vi "METIS_main_005.vi"() -> ()   [LabVIEW 2020]
uses:
  <vilib>/Analysis/1siggen.llb/Ramp Pattern by Samples.vi
  <vilib>/DAQmx/write.llb/DAQmx Write (Analog DBL 1Chan 1Samp).vi
  <vilib>/DAQmx/miscellaneous.llb/DAQmx Fill In Error Info.vi
  <vilib>/DAQmx/create/channels.llb/DAQmx Create Channel (AO-Voltage-Basic).vi
  <userlib>/caLab/Private/Get_PV.vi
  <userlib>/caLab/Private/Put_I32-1D_PV-1D.vi
  <userlib>/caLab/Private/Put_I32_PV.vi
  <userlib>/caLab/Private/Put_DBL_PV.vi
  libraries/Newport ESP301/Newport ESP301.lvlib
  <vilib>/Analysis/NI_AALBase.lvlib
  <vilib>/ptbypt/NI_PtbyPt.lvlib
  libraries/ZaberTSeries/ZaberTSeries.lvlib
  <vilib>/Analysis/NI_AALPro.lvlib
  <vilib>/Utility/file.llb/Write Delimited Spreadsheet (string).vi
  <vilib>/Analysis/1siggen.llb/Ramp Pattern by Delta.vi
panel:
  out "String":string
  out "Waveform Chart":dbl(graph)
  in  "Tab Control":T1(tab)
  in  "delay_go":bool
  in  "delay_destination_fs":dbl=0.1 caption="Destination [fs]" step=1.0 format="%#.0f"
  in  "delay_destination_mm":dbl=0.1 caption="Destination [mm]"
  in  "delay_velocity":dbl caption="velocity [mm/s]"
  in  "delay_set_vel":bool
  in  "time_zero":dbl=1.0 caption="t0 [mm]"
  out "delay_pos_mm":dbl=1.0624 caption="Position [mm]" format="%08.4g"
  out "delay_pos_fs":dbl=416.2879908072938 caption="Time [fs]"
  in  "delay_set_t0":bool
  in  "delay_rel_mm_+":bool
  in  "delay_rel_mm_-":bool
  in  "delay_stepsize_mm":dbl=1.0 caption="step size [mm]"
  in  "delay_stepsize_fs":dbl=1.0 caption="step size [fs]"
  in  "delay_rel_fs_+":bool
  in  "delay_rel_fs_-":bool
  in  "pump_rel_+":bool
  in  "pump_rel_-":bool
  in  "pump_rel_delta":dbl=1.0 caption="step size [deg]"
  out "pump_position":dbl=1.0624 caption="Position [deg]"
  in  "probe_rel_+":bool
  in  "probe_rel_-":bool
  in  "probe_rel_delta":dbl=1.0 caption="step size [deg]"
  out "probe_position":dbl=416.2879908072938 caption="Position [deg]"
  out "zaber_Ypos":i32=2950 caption="Y"
  out "zaber_Xpos":i32=1955 caption="X"
  in  "mirr_rel":i32=1 caption="relative [steps]"
  in  "mirr_Y-":bool
  in  "mirr_Y+":bool
  in  "mirr_X+":bool
  in  "mirr_X-":bool
  in  "update_scale":bool
  in  "stop after":bool
  out "scan progress":dbl(slide) scale=0.0..1.0
  in  "delay_mode_select":enum32{"Discrete Scan", "Continous Scan"}(tab)
  in  "discr_scan_MRC?":bool caption="use MRC?"
  in  "delay_waypoints":string[][](table)
  in  "delay_speedpoints":string[][](table)
  in  "stop now":bool
  in  "start":bool
  in  "Scan Axis":T2(radio)
  out "Intensity Graph":dbl[][](graph)
  out "Ydata":cluster{"Ramp Pattern":dbl[], dbl[]}[](graph)
  in  "gauss_fit":bool
  out "center":dbl
  out "FWHM":dbl
  in  "center_cursors":bool
  in  "delay_set_t0 gauss":bool
  out "current parameter value [fs | deg | steps]":dbl
  out "i":i32 caption="current iteration"
  out "current exposure time":dbl
  in  "ADC Bit/Volt":dbl=627.0
  in  "zaber_patch":u8[](array[numeric])=[0, 1]
  in  "ESP Patch":i32[](array[numeric])=[3, 2, 1] min=1 max=3 step=1
  in  "ESP301 COM PORT":refnum<visa-resource-name>="COM5"
  in  "Serial Link (RS232)":enum16{"RS232", "USB"}(ring)
  in  "toADC":tag="Dev1/ao1"
  out "ESP error":errorcluster={"status"=TRUE, "code"=-1073807339, "source"="VISA Read in Newport ESP301.lvlib:Write Command and Read.vi->Newport ESP301.lvlib:Error Query.vi->Newport ESP301.lvlib:Initialize.vi->METIS_main_004.vi"}
  out "DAC error":errorcluster={"status"=TRUE, "code"=-200220, "source"="DAQmx Create Channel (AO-Voltage-Basic).vi:1870002<append>\n<B>Device Specified: </B>Dev3\n<B>Suggested Device(s): </B>Dev1\n\n<B>Task Name: </B>_unnamedTask<2>"}
  out "DAC_Voutput":dbl=5.25341140860948 caption="output voltage"
  in  "toMRC":tag="Dev1/ao0"
  in  "zaber_VISA":refnum<visa-resource-name>="COM7"
  out "zaber_error":errorcluster
  in  "main_close":bool
  # "Pump Waveplate"
  # "Delaystage"
  # "Zaber Mirror"
  # "Probe Waveplate"
  # "Delaystage"
  # "Pump Waveplate"
  # "Probe Waveplate"
  # "X"
  # "Y"
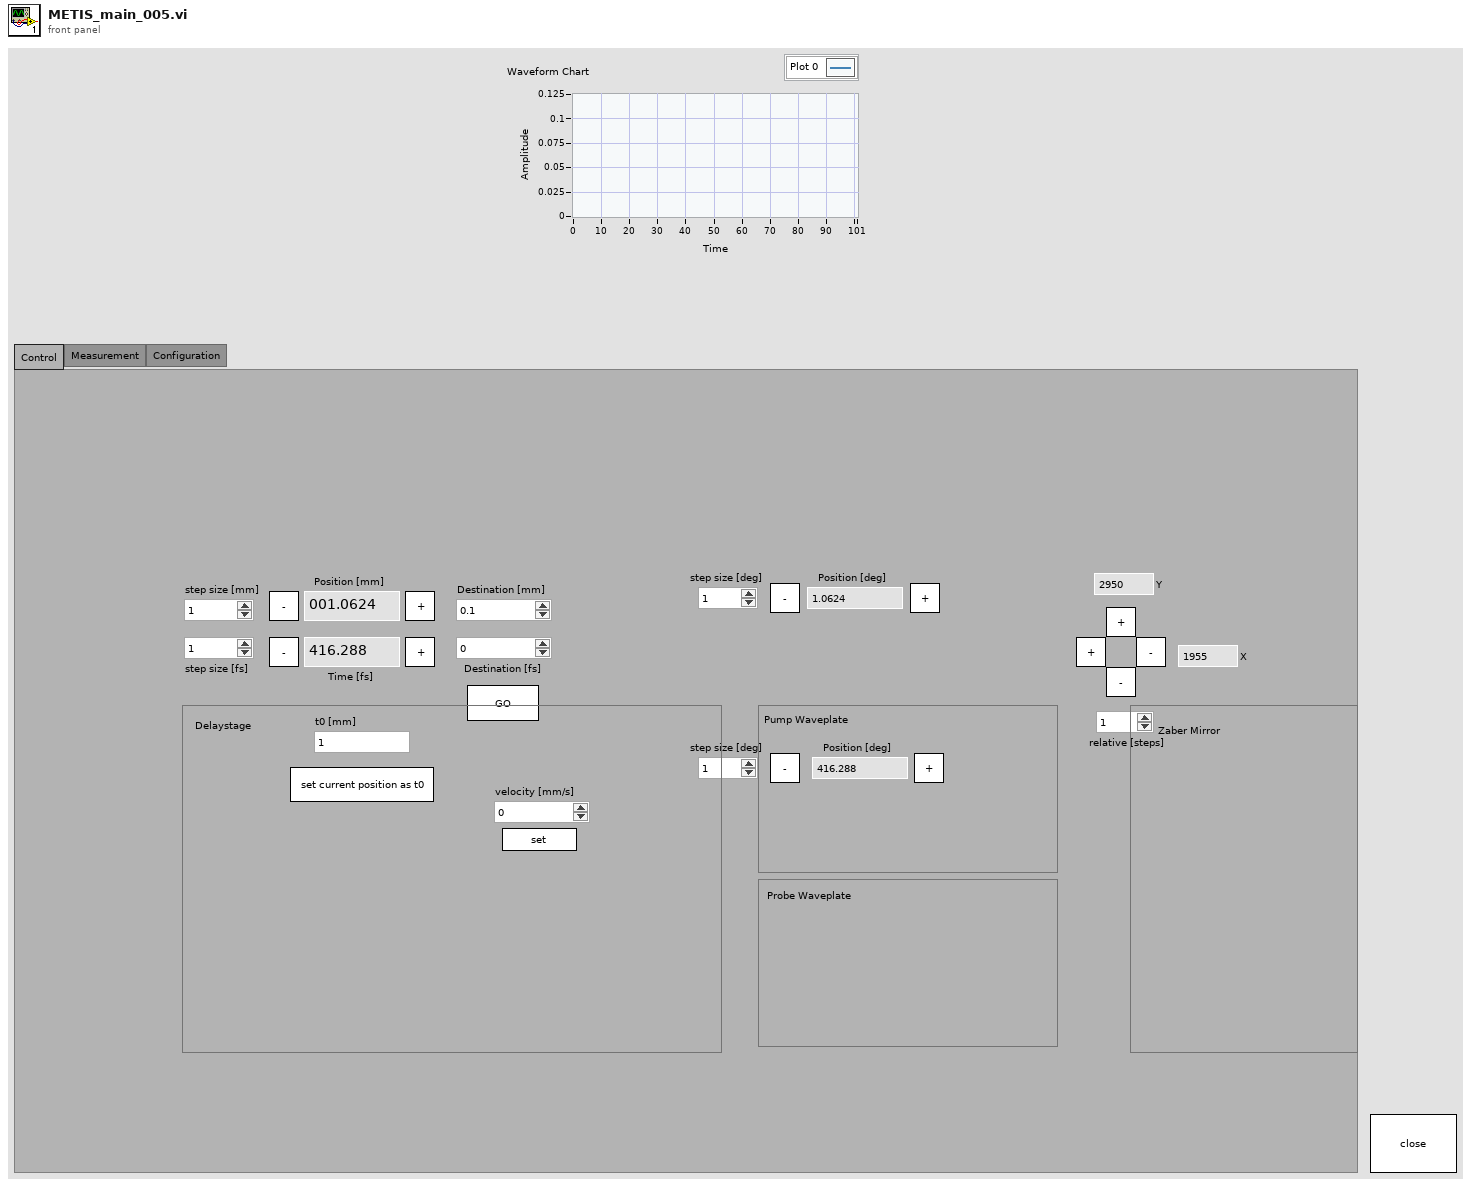
[diagram p1: front panel]
types:
  T1 = enum32{"Control", "Measurement", "Configuration"}
  T2 = enum32{"Item 0", "Item 1", "Radio Selection 3", "Radio Selection 4", "Radio Selection 5"}
  T3 = cluster{"ESP_cmd":refnum<queue>, "DAC_cmd":refnum<queue>, "meas_cmd":refnum<queue>, "zaber_cmd":refnum<queue>}
  T4 = cluster{"ESP_data":refnum<queue>, "dev2_data":refnum<queue>}
  T5 = cluster{"Axis 1":dbl, "Axis 2":dbl, "Axis 3":dbl}
  T6 = typedef "LVCursorListTypeDef.ctl" = cluster{"Name":string, "Color":u32, "Style":u8, "Point Style":u8, "Name Visible":bool, "Allow Drag":bool, "Cursor Mode":u32, "Plot":i32, "Index":i32, "Position":cluster{"X":dbl, "Y":dbl}, "X Scale":u32, "Y Scale":u32, "Watch Plots":i32[], "Watch All Plots":bool, "Plot Area":i32, "Label Offset":cluster{"X":dbl, "Y":dbl}}[]
  T7 = cluster{"Name":string, "Color":u32, "Style":u8, "Point Style":u8, "Name Visible":bool, "Allow Drag":bool, "Cursor Mode":u32, "Plot":i32, "Index":i32, "Position":cluster{"X":dbl, "Y":dbl}, "X Scale":u32, "Y Scale":u32, "Watch Plots":i32[], "Watch All Plots":bool, "Plot Area":i32, "Label Offset":cluster{"X":dbl, "Y":dbl}}
  T8 = cluster{"Name":string, "Color":u32, "Style":u8, "Point Style":u8, "Name Visible":bool, "Allow Drag":bool, "Cursor Mode":u32, "Plot":i32, "Index":i32, "Position":cluster{"X":dbl, "Y":dbl}, "X Scale":u32, "Y Scale":u32, "Watch Plots":i32[], "Watch All Plots":bool, "Plot Area":i32, "Label Offset":cluster{"X":dbl, "Y":dbl}}[]
  T9 = cluster{"Axis1 moving":bool, "Axis2 moving":bool, "Axis3 moving":bool, "Axis4 moving":bool, "Motor Power of at least one axis":bool, "Reserved":bool, "Reserved":bool, "Reserved":bool, "Axis5 moving 2":bool, "Axis6 moving 2":bool, "Reserved":bool, "Reserved":bool, "Motor Power of at least one axis":bool, "Reserved":bool, "Reserved":bool, "Reserved":bool}
  T10 = cluster{"Position (units)":dbl, "Position (units)":dbl, "Position (units)":dbl}
  T11 = cluster{"mirr_X# 4":u8, "Command":u8, dbl, "Response Count":i32}
  T12 = cluster{"mirr_X# 4":u8, "Command":u8, i32, "Response Count":i32}
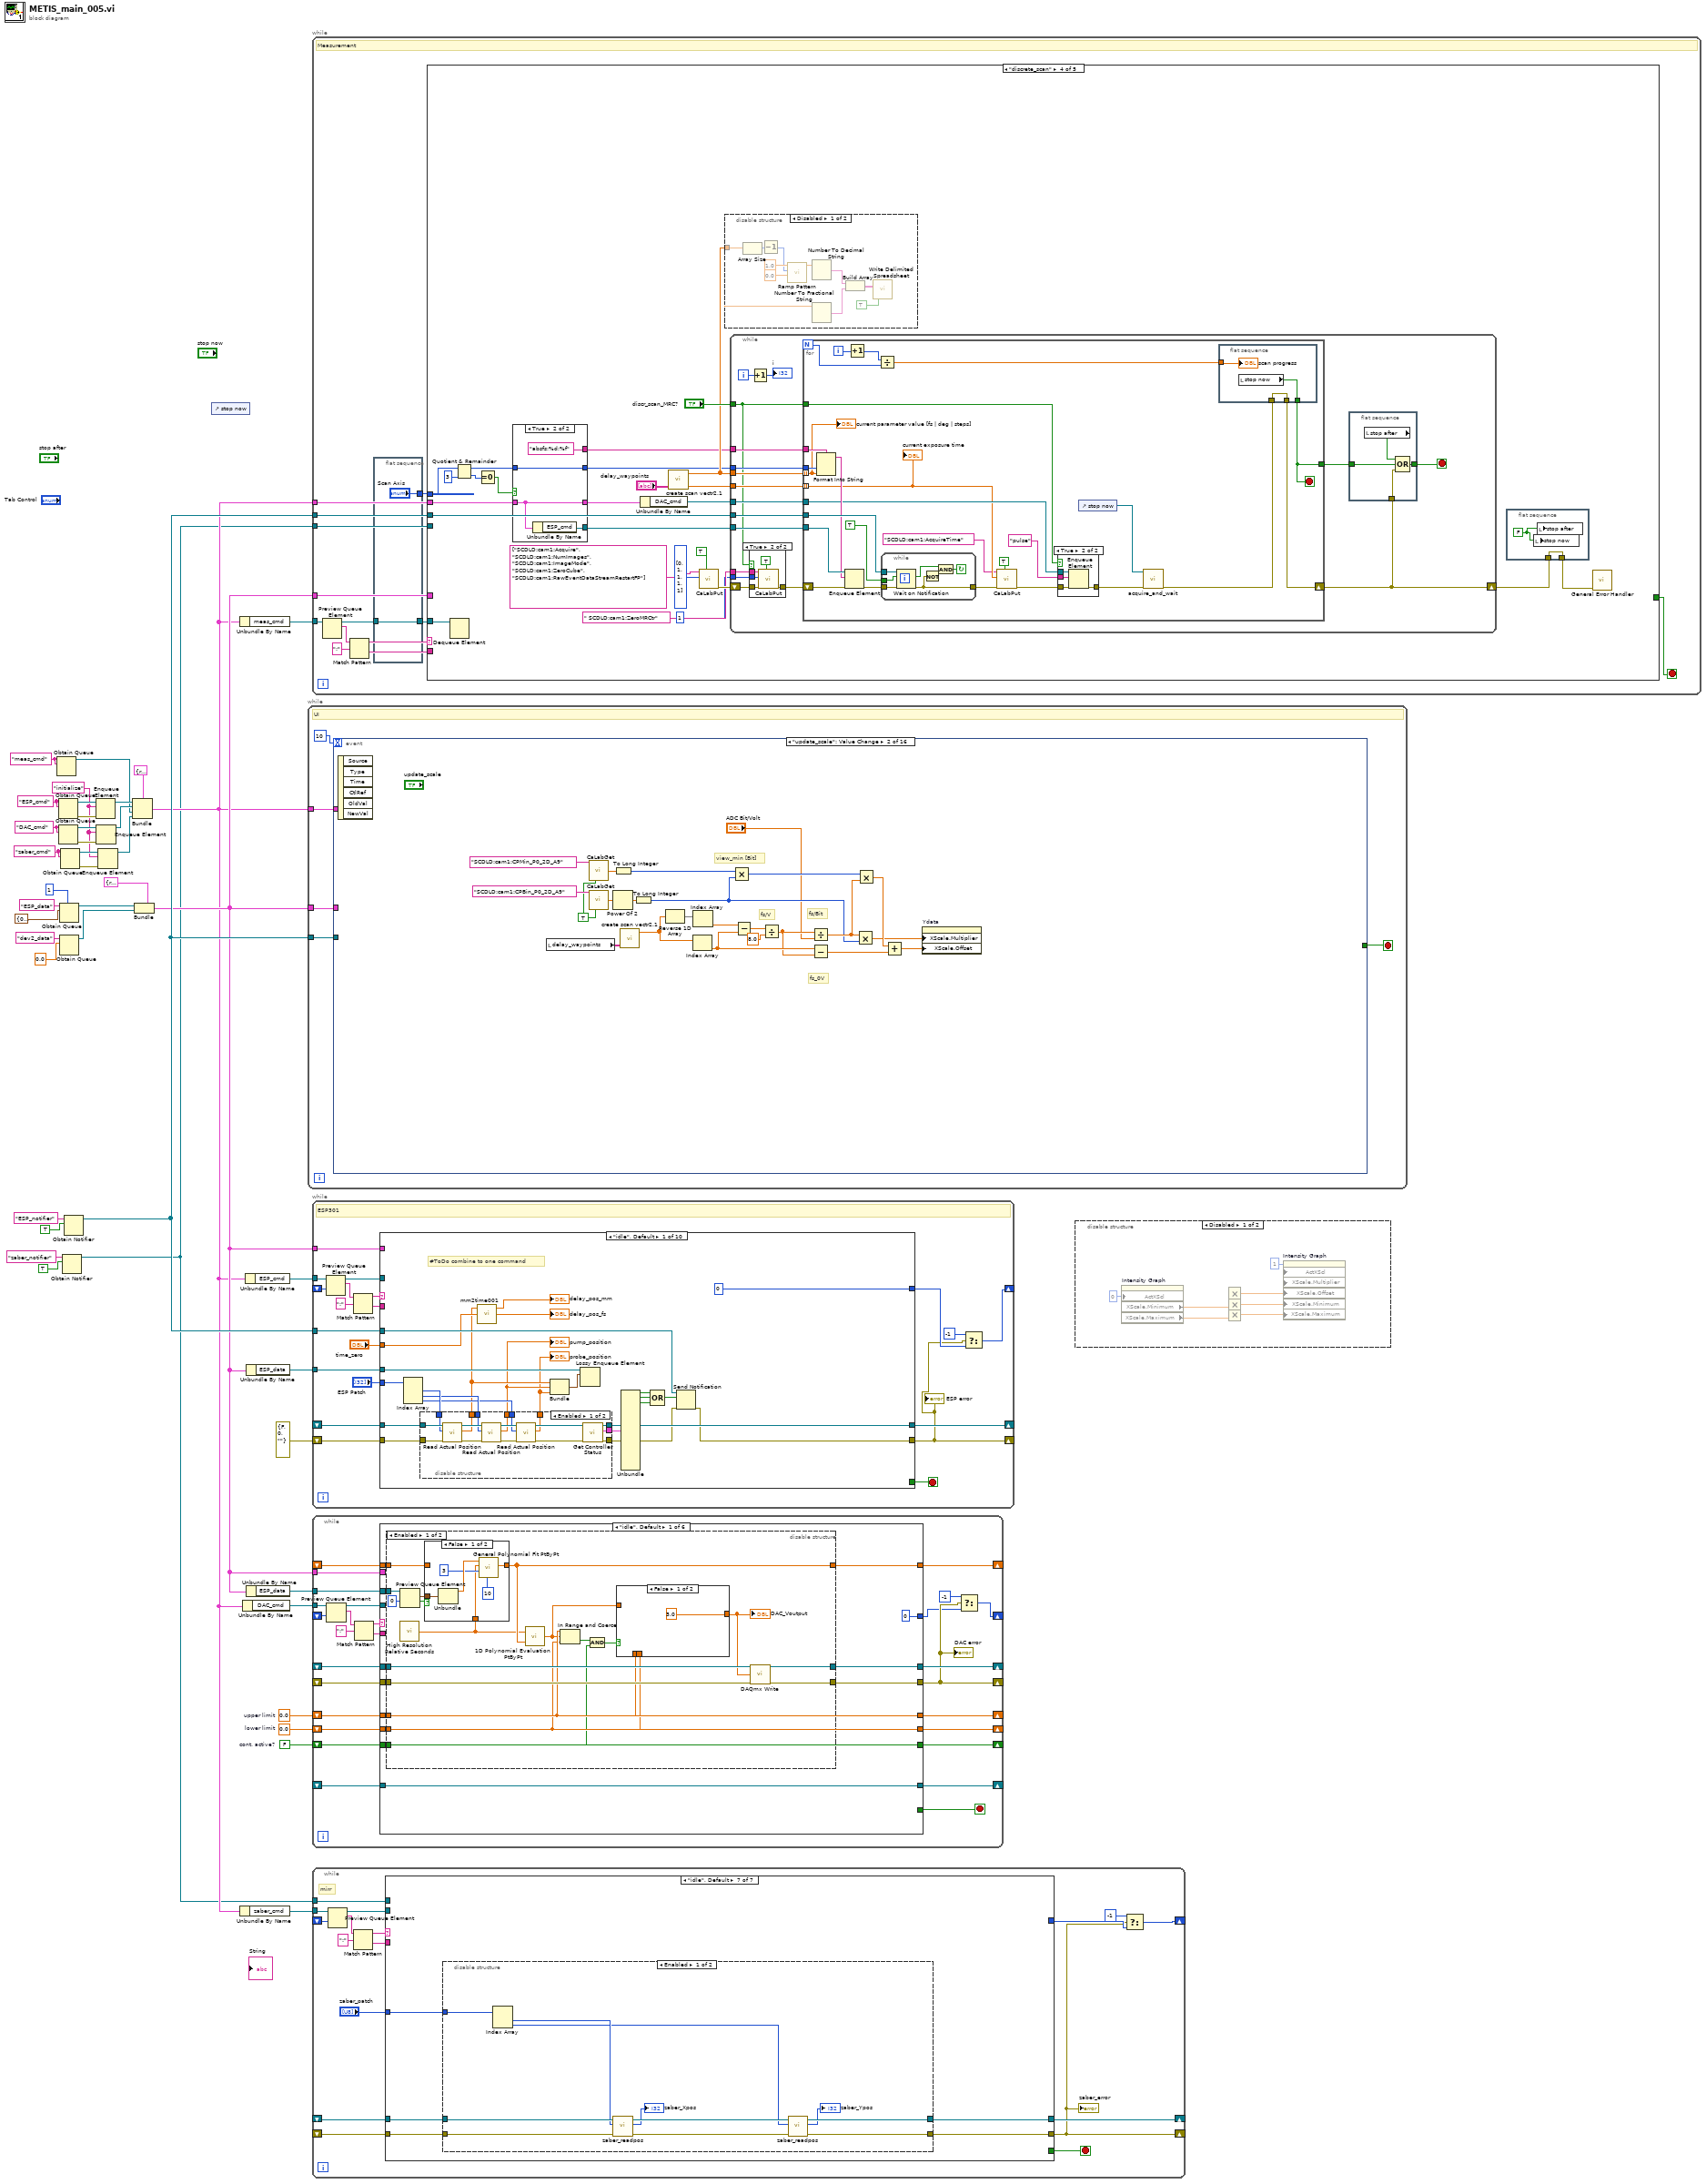
[diagram p0: block diagram]
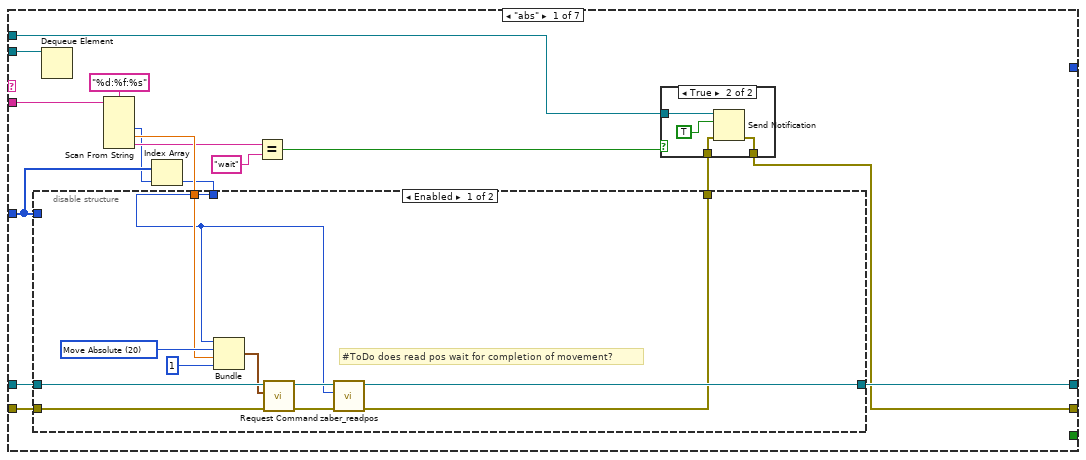
[diagram p3: hidden frame]
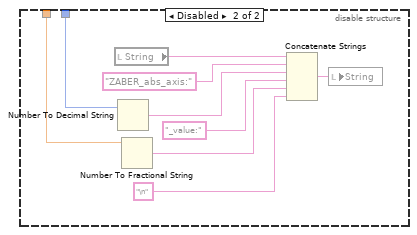
[diagram p5: hidden frame]
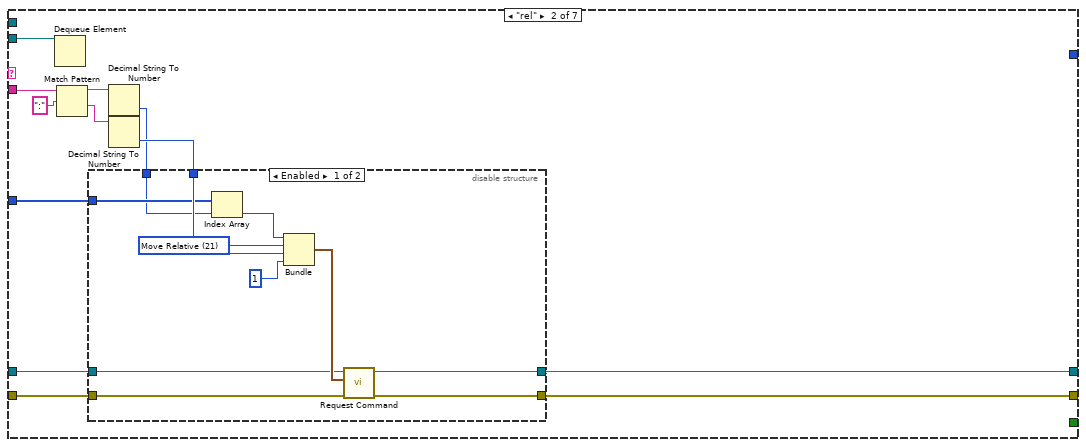
[diagram p6: hidden frame]
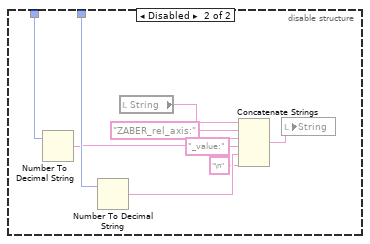
[diagram p7: hidden frame]
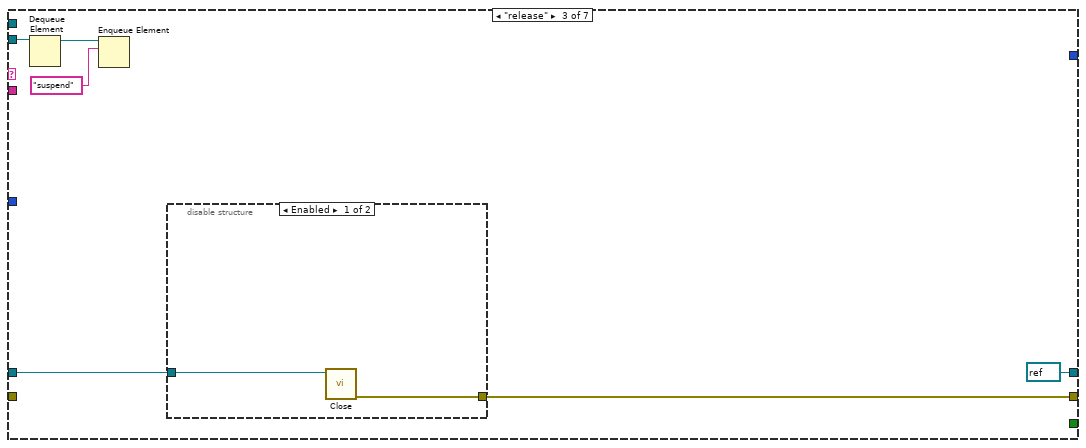
[diagram p8: hidden frame]
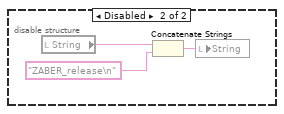
[diagram p9: hidden frame]
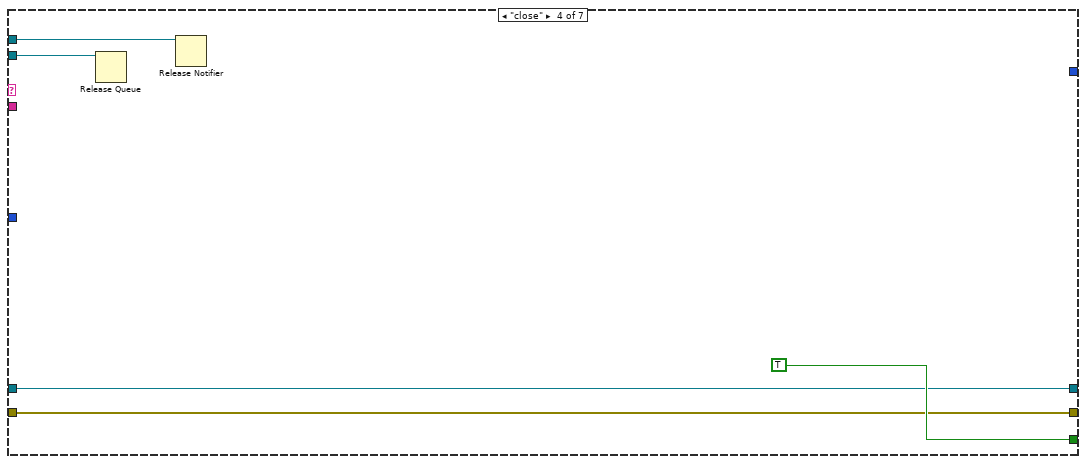
[diagram p10: hidden frame]
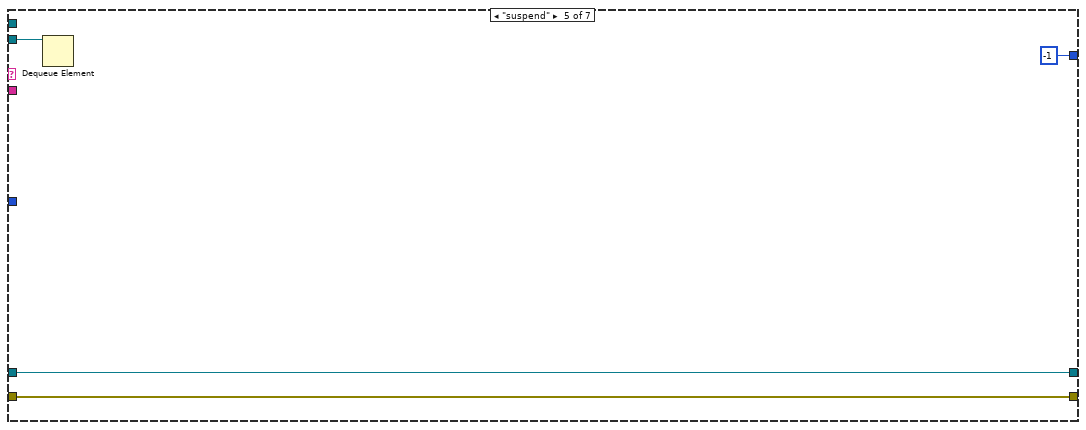
[diagram p11: hidden frame]
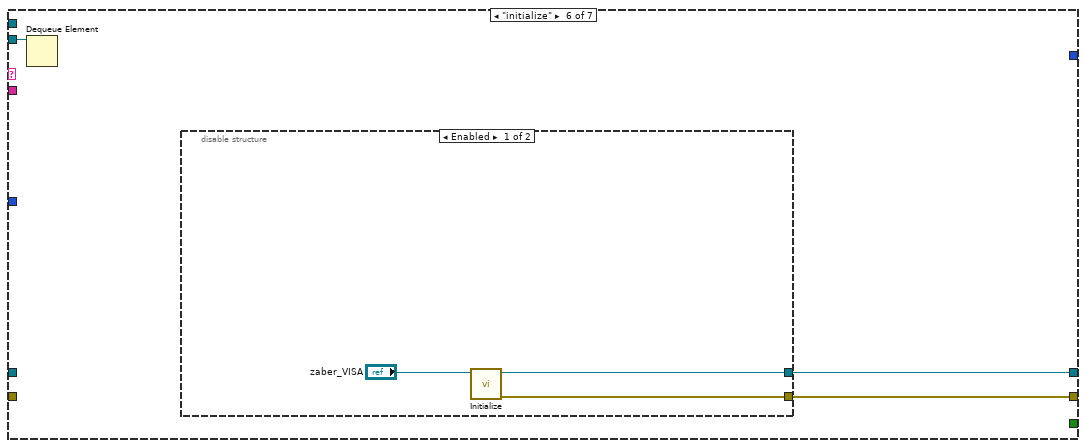
[diagram p12: hidden frame]
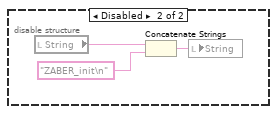
[diagram p13: hidden frame]
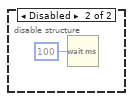
[diagram p14: hidden frame]
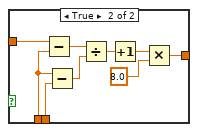
[diagram p16: hidden frame]
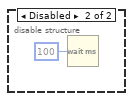
[diagram p17: hidden frame]
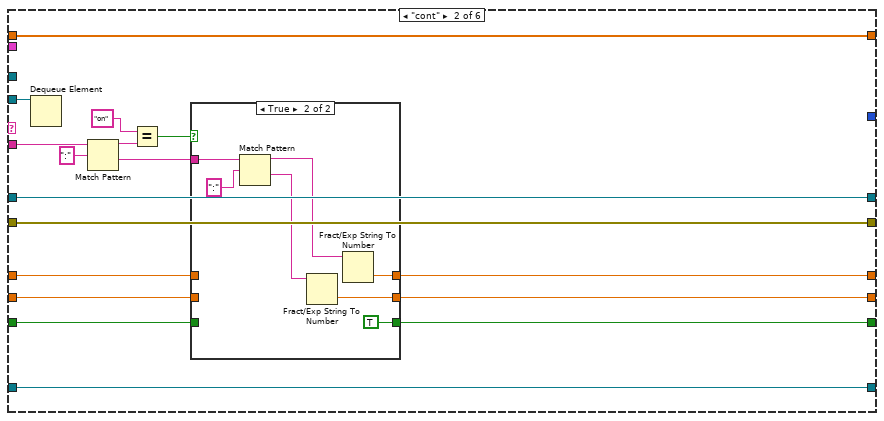
[diagram p18: hidden frame]
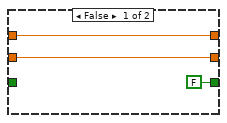
[diagram p19: hidden frame]
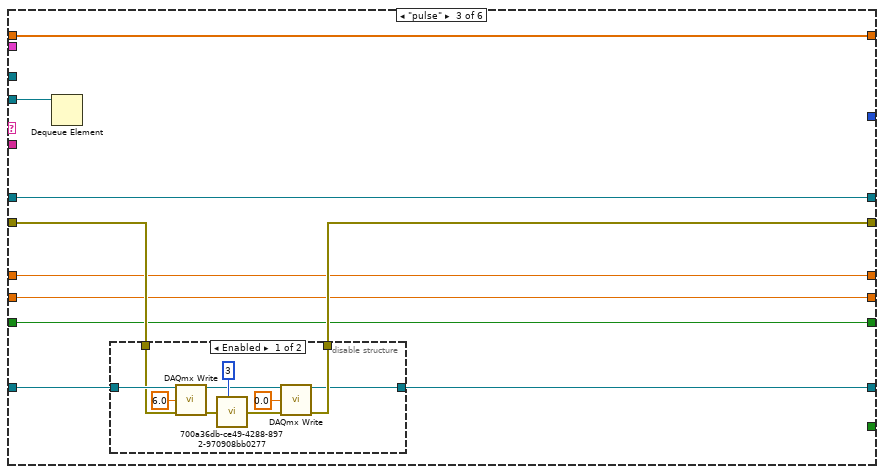
[diagram p20: hidden frame]
diagram:
  w7 = "zaber_cmd" ("name (unnamed)")
  w11 = "meas_cmd" ("name (unnamed)")
  w18 = "DAC_cmd" ("name (unnamed)")
  w3 = "initialize" ("element")
  w19 = "ESP_cmd" ("name (unnamed)")
  w32 = FALSE  # cont. active?
  w33 = 0.0  # lower limit
  w34 = 0.0  # upper limit
  n1 = Obtain Queue(name (unnamed)=w11, element data type=w11) -> (queue out=w10:refnum<queue>)  [unwired: 3 in, 2 out]
  n2 = Obtain Queue(name (unnamed)=w19, element data type=w19) -> (queue out=w28:refnum<queue>, error out=w27:errorcluster)  [unwired: 3 in, 1 out]
  n3 = Obtain Queue(name (unnamed)=w18, element data type=w18) -> (queue out=w23:refnum<queue>, error out=w24:errorcluster)  [unwired: 3 in, 1 out]
  n4 = Obtain Queue(max queue size (-1, unlimited)=1, name (unnamed)="ESP_data", element data type=T5 {"Axis 1"=0.0, "Axis 2"=0.0, "Axis 3"=0.0}) -> (queue out=w16:refnum<queue>)  [unwired: 2 in, 2 out]
  n5 = Obtain Queue(name (unnamed)="dev2_data", element data type=0.0) -> (queue out=w15:refnum<queue>)  [unwired: 3 in, 2 out]
  n6 = Obtain Queue(name (unnamed)=w7, element data type=w7) -> (queue out=w6:refnum<queue>, error out=w5:errorcluster)  [unwired: 3 in, 1 out]
  n7 = Obtain Notifier(name (unnamed)="zaber_notifier", notification data type=TRUE) -> (notifier out=w29:refnum<notifier>)  [unwired: 2 in, 2 out]
  n8 = Obtain Notifier(name (unnamed)="ESP_notifier", notification data type=TRUE) -> (notifier out=w39:refnum<notifier>)  [unwired: 2 in, 2 out]
  n9 = Enqueue Element(queue=w28, element=w3, error in (no error)=w27) -> (queue out=w25:refnum<queue>)  [unwired: 1 in, 2 out]
  n10 = Enqueue Element(queue=w23, element=w3, error in (no error)=w24) -> (queue out=w22:refnum<queue>)  [unwired: 1 in, 2 out]
  n11 = Enqueue Element(queue=w6, element=w3, error in (no error)=w5) -> (queue out=w4:refnum<queue>)  [unwired: 1 in, 2 out]
  n12 = Bundle(cluster=T3 {"ESP_cmd"=refnum, "DAC_cmd"=refnum, "meas_cmd"=refnum, "zaber_cmd"=refnum}, "ESP_cmd"=w25, "DAC_cmd"=w22, "meas_cmd"=w10, "zaber_cmd"=w4) -> (w31:T3)
  n13 = Bundle(cluster=T4 {"ESP_data"=refnum, "dev2_data"=refnum}, "ESP_data"=w16, "dev2_data"=w15) -> (w35:T4)
  n14 = control-ref of="stop now"() -> ()  [unwired: 1 out]
  n15 = Unbundle By Name(w31) -> ("meas_cmd"=w40:refnum<queue>)
  n16 = Unbundle By Name(w31) -> ("zaber_cmd"=w30:refnum<queue>)
  n17 = Unbundle By Name(w31) -> ("DAC_cmd"=w38:refnum<queue>)
  n18 = Unbundle By Name(w31) -> ("ESP_cmd"=w42:refnum<queue>)
  n19 = Unbundle By Name(w35) -> ("ESP_data"=w36:refnum<queue>)
  n20 = Unbundle By Name(w35) -> ("ESP_data"=w37:refnum<queue>)
  n21 = while {
    tunnel: w31 -> [w47]
    tunnel: w35 -> [w46]
    tunnel: w39 -> [w44]
    stop <- w45 stop-if-true
    # "UI"
    n22 = event shown="[1] \"update_scale\": Value Change" {
      selector: _ -> [_ _ _ _ _ _ _ _ _ _ _ _ _ _ _ _]
      dyn-events: _ -> [_ _ _ _ _ _ _ _ _ _ _ _ _ _ _ _]
      timeout: 10 -> [_ _ _ _ _ _ _ _ _ _ _ _ _ _ _ _]
      tunnel: w47 -> [_ _ w148 w153 _ _ _ w179 w187 w197 w207 _ w213 w223 _ w246]
      tunnel: w46 -> [_ _ _ _ _ _ _ _ _ _ _ _ _ _ _ _]
      tunnel: [_ _ _ _ _ _ _ _ _ _ _ _ _ _ _ TRUE] -> w45
      tunnel: w44 -> [_ _ _ _ _ _ _ _ _ _ _ _ _ _ _ _]
      event Timeout {
        n23 = event-data() -> ()  [unwired: 1 in, 1 out]
        n24 = disable-structure shown="Enabled" {
          frame Enabled {
            w50 = TRUE ("exclude end?")
            w63 = 0
            w81 = FALSE ("NoMDEL(F)")
            n25 = property on="Intensity Graph" class="IntGraph (strict)"() -> ("CrsrLis"=w80:T6)  [unwired: 2 in, 2 out]
            n26 = shared-variable "My Computer\\client lib.lvlib\\CPProjectionData"() -> (w48:dbl[])  [unwired: 1 in, 1 out]
            n27 = Index Array(array=w80) -> (element #1=w79:T7, element #2=w78:T7)  [unwired: 2 in]
            n28 = Unbundle By Name(w79) -> ("Position.X"=w77:dbl, "Position.Y"=w76:dbl)
            n29 = Unbundle By Name(w78) -> ("Position.X"=w74:dbl, "Position.Y"=w75:dbl)
            n30 = To Long Integer(number=w77) -> (32bit integer=w73:i32)
            n31 = To Long Integer(number=w76) -> (32bit integer=w71:i32)
            n32 = To Long Integer(number=w74) -> (32bit integer=w72:i32)
            n33 = To Long Integer(number=w75) -> (32bit integer=w70:i32)
            n34 = call-poly <userlib>:"CaLabGet.vi"("PV Name"="SCDLD:cam1:CPSize_P0_2D_A2", "NoMDEL(F)"=w81) -> ("1rst Value (number)"=w82:dbl)  [unwired: 7 in, 6 out]
            n35 = call-poly <userlib>:"CaLabGet.vi"("PV Name"="SCDLD:cam1:CPSize_P0_2D_A9", "NoMDEL(F)"=w81) -> ("1rst Value (number)"=w83:dbl)  [unwired: 7 in, 6 out]
            n36 = Build Array(w73, w72) -> (w69:i32[])
            n37 = Build Array(w71, w70) -> (w68:i32[])
            n38 = Array Max & Min(array=w69) -> (max value=w67:i32, min value=w66:i32)  [unwired: 2 out]
            n39 = Array Max & Min(array=w68) -> (max value=w65:i32, min value=w64:i32)  [unwired: 2 out]
            n40 = To Long Integer(number=w82) -> (32bit integer=w53:i32)
            n41 = To Long Integer(number=w83) -> (32bit integer=w52:i32)
            n42 = In Range and Coerce(upper limit=w52, x=w67, lower limit=w63) -> (coerced(x)=w51:i32)  [unwired: 1 out]
            n43 = In Range and Coerce(upper limit=w52, x=w66, lower limit=w63) -> (coerced(x)=w56:i32)  [unwired: 1 out]
            n44 = In Range and Coerce(upper limit=w53, x=w65, lower limit=w63) -> (coerced(x)=w61:i32)  [unwired: 1 out]
            n45 = In Range and Coerce(upper limit=w53, x=w64, lower limit=w63) -> (coerced(x)=w60:i32)  [unwired: 1 out]
            n46 = Reshape Array(w48, w53, w52) -> (w87:dbl[][])
            n47 = Transpose 2D Array(2D array=w87) -> (transposed array=w54:dbl[][])
            "Intensity Graph" <- w54
            n48 = Subtract(x=w51, y=w56) -> (x-y=w57:i32)
            n49 = Subtract(x=w61, y=w60) -> (x-y=w62:i32)
            n50 = call-poly <vilib>:"Ramp Pattern.vi"("exclude end?"=w50, "start"=w56, "end"=w51, "samples"=w57) -> ("Ramp Pattern"=w59:dbl[])  [unwired: 6 in, 1 out]
            n51 = Array Subset(array=w54, index (row)=w56, length (row)=w57, index (col)=w60, length (col)=w62) -> (w86:dbl[][])
            n52 = for {
              tunnel: w86 -> [w116] mode=indexing
              tunnel: [w115] -> w58 mode=indexing
              n53 = Add Array Elements(numeric array=w116) -> (sum=w115:dbl)
            }
            n54 = case shown="True" "gauss_fit" {
              tunnel: w59 -> [_ w109]
              tunnel: w58 -> [_ w108]
              tunnel: w56 -> [_ w107]
              tunnel: [cluster{"Ramp Pattern":dbl[], dbl[]} {"Ramp Pattern"=[], []} w102] -> w55
              tunnel: w51 -> [_ w99]
              tunnel: w50 -> [_ w98]
              frame False {
              }
              frame True {
                n55 = Decrement(x=w99) -> (x-1=w100:i32)
                n56 = property on="Ydata" class="XYGraph (strict)"() -> ("XScale.Multiplier"=w92:dbl, "XScale.Offset"=w95:dbl)  [unwired: 2 in, 2 out]
                n57 = call-poly <vilib>:"Ramp Pattern.vi"("exclude end?"=w98, "start"=w107, "end"=w100, "samples"=1000) -> ("Ramp Pattern"=w105:dbl[])  [unwired: 6 in, 1 out]
                n58 = call <vilib>:"Gaussian Peak Fit.vi"("Y"=w108, "X"=w109) -> ("amplitude"=w104:dbl, "center"=w97:dbl, "standard deviation"=w101:dbl)  [unwired: 7 in, 4 out]
                n59 = Multiply(x=w97, y=w92) -> (x*y=w96:dbl)
                n60 = call "std2fwhm.vi"("std. dev."=w101) -> ("FWHM"=w93:dbl)
                n61 = Add(x=w96, y=w95) -> (x+y=→"center":dbl)
                n62 = Multiply(x=w93, y=w92) -> (x*y=→"FWHM":dbl)
                n63 = for {
                  tunnel: w105 -> [w114] mode=indexing
                  tunnel: w101 -> [w113]
                  tunnel: w97 -> [w112]
                  tunnel: [w111] -> w103 mode=indexing
                  tunnel: w104 -> [w110]
                  n64 = call "gauss.vi"("X"=w114, "amplitude"=w110, "center"=w112, "std. dev."=w113) -> ("y"=w111:dbl)
                }
                n65 = Bundle("Ramp Pattern"=w105, w103) -> (w102:cluster{"Ramp Pattern":dbl[], dbl[]})  [unwired: 1 in]
              }
            }
            n66 = Bundle("Ramp Pattern"=w59, w58) -> (w85:cluster{"Ramp Pattern":dbl[], dbl[]})  [unwired: 1 in]
            n67 = Build Array(w85, w55) -> (→"Ydata":cluster{"Ramp Pattern":dbl[], dbl[]}[])
          }
          frame Disabled {
          }
        }
        n68 = disable-structure shown="Disabled" {
          frame Disabled {
            n69 = while {
              shift-right: [w120] -> _
              shift-left: _ -> [w119]
              stop <- TRUE stop-if-true
              n70 = call <vilib>:"High Resolution Relative Seconds.vi"() -> ("relative seconds"=w120:dbl)
              n71 = Subtract(x=w120, y=w119) -> (x-y=w118:dbl)
              n72 = Reciprocal(x=w118) -> (1/x=→"Waveform Chart":dbl)
            }
          }
          frame Enabled {
          }
        }
      }
      event "update_scale": Value Change {
        w124 = TRUE ("NoMDEL(F)")
        # "fs/Bit"
        # "fs_0V"
        # "view_min [Bit]"
        # "fs/V"
        n73 = event-data() -> ()  [unwired: 1 in, 6 out]
        n74 = local read "delay_waypoints"() -> (w129:string[][])
        n75 = call-poly <userlib>:"CaLabGet.vi"("PV Name"="SCDLD:cam1:CPMin_P0_2D_A9", "NoMDEL(F)"=w124) -> ("1rst Value (number)"=w139:dbl)  [unwired: 7 in, 6 out]
        n76 = call-poly <userlib>:"CaLabGet.vi"("PV Name"="SCDLD:cam1:CPBin_P0_2D_A9", "NoMDEL(F)"=w124) -> ("1rst Value (number)"=w141:dbl)  [unwired: 7 in, 6 out]
        n77 = Power Of 2(x=w141) -> (2^x=w140:dbl)
        n78 = To Long Integer(number=w139) -> (32bit integer=w123:i32)
        n79 = call "create scan vectr2.1.vi"("Table Control"=w129) -> ("positions"=w128:dbl[])  [unwired: 3 in, 1 out]
        n80 = To Long Integer(number=w140) -> (32bit integer=w132:i32)
        n81 = Reverse 1D Array(array=w128) -> (reversed array=w144:dbl[])
        n82 = Index Array(array=w128) -> (element=w138:dbl)  [unwired: 1 in]
        n83 = Index Array(array=w144) -> (element=w143:dbl)  [unwired: 1 in]
        n84 = Multiply(x=w123, y=w132) -> (x*y=w136:i32)
        n85 = Subtract(x=w143, y=w138) -> (x-y=w142:dbl)
        n86 = Divide(x=w142, y=8.0) -> (x/y=w137:dbl)
        n87 = Divide(x=w137, y="ADC Bit/Volt") -> (x/y=w133:dbl)
        n88 = Subtract(x=w138, y=w137) -> (x-y=w135:dbl)
        n89 = Multiply(x=w133, y=w132) -> (x*y=w131:dbl)
        n90 = Multiply(x=w136, y=w133) -> (x*y=w134:dbl)
        n91 = Add(x=w134, y=w135) -> (x+y=w130:dbl)
        n92 = property on="Ydata" class="XYGraph (strict)"("XScale.Multiplier"=w131, "XScale.Offset"=w130) -> ()  [unwired: 2 in, 2 out]
      }
      event "start": Value Change {
        n93 = event-data() -> ()  [unwired: 1 in, 1 out]
        n94 = case shown="\"Continous Scan\"" "delay_mode_select" {
          tunnel: ["discrete_scan" ("string") "cont_scan" ("string")] -> w145
          frame "Discrete Scan", Default {
          }
          frame "Continous Scan" {
          }
        }
        n95 = Unbundle By Name(w148) -> ("meas_cmd"=w149:refnum<queue>)
        n96 = local write "scan progress"(0.0 ("scan progress")) -> ()
        n97 = Enqueue Element(queue=w149, element=w145) -> ()  [unwired: 2 in, 3 out]
      }
      event "mirr_Y-", "mirr_Y+", "mirr_X+", "mirr_X-": Value Change {
        n98 = event-data() -> ()  [unwired: 1 in, 1 out]
        n99 = Unbundle By Name(w153) -> ("zaber_cmd"=w152:refnum<queue>)
        n100 = Or(x="mirr_X+", y="mirr_X-") -> (x .or. y?=w163:bool)
        n101 = Or(x="mirr_X-", y="mirr_Y-") -> (x .or. y?=w169:bool)
        n102 = Negate(x="mirr_rel") -> (-x=w168:i32)
        n103 = Select(t=0, s=w163, f=1) -> (s? t:f=w162:i32)
        n104 = Select(t=w168, s=w169, f="mirr_rel") -> (s? t:f=w160:i32)
        n105 = Number To Decimal String(number=w162) -> (decimal integer string=w161:string)  [unwired: 1 in]
        n106 = Number To Decimal String(number=w160) -> (decimal integer string=w159:string)  [unwired: 1 in]
        n107 = Concatenate Strings("rel:" ("string"), w161, ":" ("string"), w159) -> (w158:string)
        n108 = Enqueue Element(queue=w152, element=w158) -> ()  [unwired: 2 in, 3 out]
      }
      event "delay_destination_fs": Value Change {
        n109 = event-data() -> ()  [unwired: 1 in, 6 out]
        n110 = local read "time_zero"() -> (w172:dbl)
        n111 = call "time2mm001.vi"("Offset (mm)"=w172, "time"="delay_destination_fs") -> ("position (mm)"=w171:dbl)  [unwired: 1 in]
        n112 = local write "delay_destination_mm"(w171) -> ()
      }
      event "delay_set_t0": Value Change {
        n113 = event-data() -> ()  [unwired: 1 in, 1 out]
        n114 = local read "delay_pos_mm"() -> (w173:dbl)
        n115 = local write "time_zero"(w173) -> ()
      }
      event "delay_set_t0 gauss": Value Change {
        n116 = event-data() -> ()  [unwired: 1 in, 6 out]
        n117 = local read "time_zero"() -> (w176:dbl)
        n118 = local read "center"() -> (w175:dbl)
        n119 = call "time2mm001.vi"("Offset (mm)"=w176, "time"=w175) -> ("position (mm)"=w174:dbl)  [unwired: 1 in]
        n120 = local write "time_zero"(w174) -> ()
      }
      event "delay_rel_mm_+", "delay_rel_mm_-": Value Change {
        n121 = event-data() -> ()  [unwired: 1 in, 1 out]
        n122 = Unbundle By Name(w179) -> ("ESP_cmd"=w180:refnum<queue>)
        n123 = Negate(x="delay_stepsize_mm") -> (-x=w184:dbl)
        n124 = Select(t="delay_stepsize_mm", s="delay_rel_mm_+", f=w184) -> (s? t:f=w182:dbl)
        n125 = Format Into String(format string="rel:0:%f", w182) -> (resulting string=w181:string)  [unwired: 2 in, 1 out]
        n126 = Enqueue Element(queue=w180, element=w181) -> ()  [unwired: 2 in, 3 out]
      }
      event "delay_rel_fs_+", "delay_rel_fs_-": Value Change {
        n127 = event-data() -> ()  [unwired: 1 in, 1 out]
        n128 = Unbundle By Name(w187) -> ("ESP_cmd"=w188:refnum<queue>)
        n129 = Negate(x="delay_stepsize_fs") -> (-x=w192:dbl)
        n130 = Select(t="delay_stepsize_fs", s="delay_rel_fs_+", f=w192) -> (s? t:f=w190:dbl)
        n131 = Format Into String(format string="relfs:0:%f", w190) -> (resulting string=w189:string)  [unwired: 2 in, 1 out]
        n132 = Enqueue Element(queue=w188, element=w189) -> ()  [unwired: 2 in, 3 out]
      }
      event "pump_rel_+", "pump_rel_-": Value Change {
        n133 = event-data() -> ()  [unwired: 1 in, 1 out]
        n134 = Unbundle By Name(w197) -> ("ESP_cmd"=w193:refnum<queue>)
        n135 = Negate(x="pump_rel_delta") -> (-x=w199:dbl)
        n136 = Select(t="pump_rel_delta", s="pump_rel_+", f=w199) -> (s? t:f=w195:dbl)
        n137 = Format Into String(format string="rel:1:%f", w195) -> (resulting string=w194:string)  [unwired: 2 in, 1 out]
        n138 = Enqueue Element(queue=w193, element=w194) -> ()  [unwired: 2 in, 3 out]
      }
      event "probe_rel_+", "probe_rel_-": Value Change {
        n139 = event-data() -> ()  [unwired: 1 in, 1 out]
        n140 = Unbundle By Name(w207) -> ("ESP_cmd"=w203:refnum<queue>)
        n141 = Negate(x="probe_rel_delta") -> (-x=w208:dbl)
        n142 = Select(t="probe_rel_delta", s="probe_rel_+", f=w208) -> (s? t:f=w205:dbl)
        n143 = Format Into String(format string="rel:2:%f", w205) -> (resulting string=w204:string)  [unwired: 2 in, 1 out]
        n144 = Enqueue Element(queue=w203, element=w204) -> ()  [unwired: 2 in, 3 out]
      }
      event "delay_destination_mm": Value Change {
        n145 = event-data() -> ()  [unwired: 1 in, 1 out]
        n146 = local read "time_zero"() -> (w211:dbl)
        n147 = call "mm2time001.vi"("Offset (mm)"=w211, "distance (mm)"="delay_destination_mm") -> ("time in fs"=w210:dbl)  [unwired: 1 in]
        n148 = local write "delay_destination_fs"(w210) -> ()
      }
      event "delay_set_vel": Value Change {
        n149 = event-data() -> ()  [unwired: 1 in, 2 out]
        n150 = Number To Fractional String(number="delay_velocity") -> (F-format string=w216:string)  [unwired: 3 in]
        n151 = Unbundle By Name(w213) -> ("ESP_cmd"=w217:refnum<queue>)
        n152 = Concatenate Strings("vel:0:" ("string"), w216) -> (w215:string)
        n153 = Enqueue Element(queue=w217, element=w215) -> ()  [unwired: 2 in, 3 out]
      }
      event "delay_go": Value Change {
        n154 = event-data() -> ()  [unwired: 1 in, 1 out]
        n155 = local read "delay_destination_mm"() -> (w218:dbl)
        n156 = Number To Fractional String(number=w218) -> (F-format string=w221:string)  [unwired: 3 in]
        n157 = Unbundle By Name(w223) -> ("ESP_cmd"=w222:refnum<queue>)
        n158 = Concatenate Strings("abs:0:" ("string"), w221) -> (w219:string)
        n159 = Enqueue Element(queue=w222, element=w219) -> ()  [unwired: 2 in, 3 out]
      }
      event "center_cursors": Value Change {
        w235 = 0.1 ("x")
        n160 = event-data() -> ()  [unwired: 1 in, 1 out]
        n161 = property on="Intensity Graph" class="IntGraph (strict)"("ActXScl"=0 ("Active X Scale")) -> ("XScale.Maximum"=w233:dbl, "XScale.Minimum"=w234:dbl, "YScale.Maximum"=w230:dbl, "YScale.Minimum"=w231:dbl)  [unwired: 2 in, 2 out]
        n162 = Subtract(x=w233, y=w234) -> (x-y=w237:dbl)
        n163 = Subtract(x=w230, y=w231) -> (x-y=w236:dbl)
        n164 = Multiply(x=w235, y=w237) -> (x*y=w232:dbl)
        n165 = Multiply(x=w236, y=w235) -> (x*y=w229:dbl)
        n166 = Subtract(x=w233, y=w232) -> (x-y=w226:dbl)
        n167 = Add(x=w232, y=w234) -> (x+y=w228:dbl)
        n168 = Subtract(x=w230, y=w229) -> (x-y=w225:dbl)
        n169 = Add(x=w229, y=w231) -> (x+y=w227:dbl)
        n170 = property on="Intensity Graph" class="IntGraph (strict)"() -> ("CrsrLis"=w243:T6)  [unwired: 2 in, 2 out]
        n171 = Index Array(array=w243) -> (element #1=w242:T7, element #2=w241:T7)  [unwired: 2 in]
        n172 = Bundle By Name(cluster=w242, "Position.X"=w228, "Position.Y"=w227) -> (w240:T7)
        n173 = Bundle By Name(cluster=w241, "Position.X"=w226, "Position.Y"=w225) -> (w239:T7)
        n174 = Build Array(w240, w239) -> (w238:T8)
        n175 = property on="Intensity Graph" class="IntGraph (strict)"("CrsrLis"=w238) -> ()  [unwired: 2 in, 2 out]
      }
      event "main_close": Value Change {
        n176 = event-data() -> ()  [unwired: 1 in, 1 out]
        n177 = Cluster To Array(cluster=w246) -> (array=w245:refnum<queue>[])
        n178 = for {
          tunnel: w245 -> [w251] mode=indexing
          n179 = Flush Queue(queue=w251) -> (queue out=w247:refnum<queue>)  [unwired: 1 in, 2 out]
          n180 = Enqueue Element(queue=w247, element="release") -> (queue out=w249:refnum<queue>)  [unwired: 2 in, 2 out]
          n181 = Enqueue Element(queue=w249, element="close") -> ()  [unwired: 2 in, 3 out]
        }
      }
    }
  }
  n182 = while {
    tunnel: w40 -> [w262]
    tunnel: w39 -> [w259]
    tunnel: w31 -> [w260]
    tunnel: w35 -> [w258]
    tunnel: w29 -> [w255]
    stop <- w254 stop-if-true
    # "Measurement"
    n183 = Preview Queue Element(queue=w262) -> (queue out=w253:refnum<queue>, element=w263:string)  [unwired: 2 in, 2 out]
    n184 = Match Pattern(string=w263, regular expression=":") -> (before substring=w261:string, after substring=w257:string)  [unwired: 1 in, 2 out]
    n185 = flat-sequence {
      tunnel: ["Scan Axis"] -> w256
      tunnel: w253 -> [w265]
      tunnel: [w265] -> w252
      frame #0 {
      }
    }
    n186 = case shown="\"discrete_scan\"" w261 {
      tunnel: w252 -> [w268 _ w271 w296 w418]
      tunnel: w260 -> [_ _ _ w289 w403]
      tunnel: w259 -> [_ _ _ w291 w392]
      tunnel: w258 -> [_ _ _ _ w413]
      tunnel: w257 -> [_ _ _ _ _]
      tunnel: w256 -> [_ _ _ w282 w386]
      tunnel: w255 -> [_ _ _ _ _]
      tunnel: [TRUE _ _ _ _] -> w254
      frame "close" {
        (unwired) TRUE
        n187 = Dequeue Element(queue=w268) -> (queue out=w269:refnum<queue>, error out=w270:errorcluster)  [unwired: 2 in, 2 out]
        n188 = Release Queue(queue=w269, error in (no error)=w270) -> ()  [unwired: 1 in, 3 out]
      }
      frame "idle", Default {
      }
      frame "release" {
        n189 = Dequeue Element(queue=w271) -> ()  [unwired: 2 in, 4 out]
      }
      frame "discrete_scan" {
        n190 = Dequeue Element(queue=w296) -> ()  [unwired: 2 in, 4 out]
        n191 = Quotient & Remainder(x=w282, y=3) -> (x-y*floor(x/y)=w274:u32, floor(x/y)=w280:u32)
        n192 = Equal To 0?(x=w280) -> (x = 0?=w276:bool)
        n193 = case shown="True" w276 {
          tunnel: [w310 w314] -> w290
          tunnel: w289 -> [w309 w313]
          tunnel: [w309 w313] -> w275
          tunnel: w274 -> [w308 w312]
          tunnel: [w308 w312] -> w273
          tunnel: ["abs:%d:%f:wait" ("format string") "absfs:%d:%f" ("format string")] -> w272
          frame False {
            n194 = Unbundle By Name(w309) -> ("zaber_cmd"=w310:refnum<queue>)
          }
          frame True {
            n195 = Unbundle By Name(w313) -> ("ESP_cmd"=w314:refnum<queue>)
          }
        }
        n196 = Unbundle By Name(w275) -> ("DAC_cmd"=w288:refnum<queue>)
        n197 = call "create scan vectr2.1.vi"("Table Control"="delay_waypoints") -> ("parameters"=w292:dbl[], "positions"=w277:dbl[])  [unwired: 3 in]
        n198 = call-poly <userlib>:"CaLabPut.vi"("Synchronous (F)"=TRUE, "Values"=i32[] [0, 1, 1, 1, 1], "PV Names"=string[] ["SCDLD:cam1:Acquire", "SCDLD:cam1:NumImages", "SCDLD:cam1:ImageMode", "SCDLD:cam1:ZeroCube", "SCDLD:cam1:RawEventDataStreamRestartFP"]) -> ("Error out"=w287:errorcluster)  [unwired: 5 in, 3 out]
        n199 = disable-structure shown="Disabled" {
          disable-tunnel: w277 -> [w297 _]
          frame Disabled {
            n200 = Array Size(array=w297) -> (size(s)=w300:i32)
            n201 = Decrement(x=w300) -> (x-1=w299:i32)
            n202 = call-poly <vilib>:"Ramp Pattern.vi"("start"=0.0, "end"=w299, "delta"=1.0) -> ("Ramp Pattern"=w304:dbl[])  [unwired: 6 in, 2 out]
            n203 = Number To Decimal String(number=w304) -> (decimal integer string=w303:string[])  [unwired: 1 in]
            n204 = Number To Fractional String(number=w297) -> (F-format string=w302:string[])  [unwired: 3 in]
            n205 = Build Array(w303, w302) -> (w301:string[][])
            n206 = call-poly <vilib>:"Write Delimited Spreadsheet.vi"("2D data"=w301, "transpose? (no:F)"=TRUE) -> ()  [unwired: 12 in, 2 out]
          }
          frame Enabled {
          }
        }
        n207 = while {
          tunnel: w292 -> [w333]
          tunnel: w291 -> [w332]
          tunnel: w290 -> [w331]
          tunnel: w288 -> [w330]
          tunnel: w272 -> [w329]
          tunnel: w277 -> [w328]
          tunnel: w273 -> [w327]
          tunnel: "discr_scan_MRC?" -> [w326]
          shift-right: [w320] -> w279
          shift-left: w287 -> [w325]
          tunnel: " SCDLD:cam1:ZeroMRCtr" -> [w324]
          tunnel: 1 ("Numeric") -> [w323]
          i -> [w318]
          stop <- w319 stop-if-true
          n208 = case shown="True" w326 {
            tunnel: w325 -> [w338 w343]
            tunnel: w324 -> [_ w342]
            tunnel: w323 -> [_ w341]
            tunnel: [w338 w340] -> w322
            frame False {
            }
            frame True {
              n209 = call-poly <userlib>:"CaLabPut.vi"("Synchronous (F)"=TRUE, "Error in (no error)"=w343, "Value"=w341, "PV Name"=w342) -> ("Error out"=w340:errorcluster)  [unwired: 4 in, 3 out]
            }
          }
          n210 = Increment(x=w318) -> (x+1=→"i":i32)
          n211 = for {
            N -> [w356]
            tunnel: w328 -> [w361] mode=indexing
            tunnel: w333 -> [w354] mode=indexing
            tunnel: w332 -> [w369]
            tunnel: w331 -> [w367]
            shift-right: [w359] -> w320
            shift-left: w322 -> [w368]
            tunnel: w330 -> [w364]
            tunnel: w329 -> [w363]
            tunnel: w327 -> [w362]
            tunnel: w326 -> [w358]
            tunnel: [w348] -> w321
            i -> [w347]
            stop <- w348 stop-if-true
            n212 = Format Into String(format string=w363, w362, w361) -> (resulting string=w366:string)  [unwired: 2 in, 1 out]
            n213 = Enqueue Element(queue=w367, element=w366, error in (no error)=w368) -> (error out=w365:errorcluster)  [unwired: 1 in, 2 out]
            n214 = Increment(x=w347) -> (x+1=w357:i32)
            n215 = Divide(x=w357, y=w356) -> (x/y=w355:dbl)
            n216 = while {
              tunnel: w369 -> [w384]
              tunnel: [w381] -> w353
              tunnel: w365 -> [w383]
              tunnel: TRUE ("ignore previous (F)") -> [w382]
              stop <- w378 continue-if-true
              n217 = Wait on Notification(notifier=w384, ignore previous (F)=w382, error in (no error)=w383) -> (notification=w379:bool, error out=w381:errorcluster)  [unwired: 1 in, 2 out]
              n218 = Not(x=w381) -> (.not. x?=w380:bool)
              n219 = And(x=w379, y=w380) -> (x .and. y?=w378:bool)
            }
            n220 = call-poly <userlib>:"CaLabPut.vi"("Synchronous (F)"=TRUE, "Error in (no error)"=w353, "Value"=w354, "PV Name"="SCDLD:cam1:AcquireTime") -> ("Error out"=w351:errorcluster)  [unwired: 4 in, 3 out]
            n221 = case shown="True" w358 {
              tunnel: w364 -> [_ w374]
              tunnel: [w370 w373] -> w346
              tunnel: "pulse" ("element") -> [_ w372]
              tunnel: w351 -> [w370 w371]
              frame False {
              }
              frame True {
                n222 = Enqueue Element(queue=w374, element=w372, error in (no error)=w371) -> (error out=w373:errorcluster)  [unwired: 1 in, 2 out]
              }
            }
            n223 = control-ref of="stop now"() -> (w344:refnum<vi>)
            n224 = call "acquire_and_wait.vi"("Error in (no error)"=w346, "stop now"=w344) -> ("Error out"=w345:errorcluster)  [unwired: 9 in]
            n225 = flat-sequence {
              tunnel: w345 -> [w377]
              tunnel: [w377] -> w359
              tunnel: w355 -> [w375]
              tunnel: [w376] -> w348
              frame #0 {
                n226 = local read "stop now"() -> (w376:bool)
                "scan progress" <- w375
              }
            }
            "current parameter value [fs | deg | steps]" <- w361
            "current exposure time" <- w354
          }
          n227 = flat-sequence {
            tunnel: w321 -> [w337]
            tunnel: w320 -> [w336]
            tunnel: [w335] -> w319
            frame #0 {
              n228 = local read "stop after"() -> (w334:bool)
              n229 = Compound Arithmetic op=OR(w334, w337, w336) -> (w335:bool)
            }
          }
        }
        n230 = flat-sequence {
          tunnel: w279 -> [w316]
          tunnel: [w316] -> w278
          frame #0 {
            w315 = FALSE
            n231 = local write "stop now"(w315) -> ()
            n232 = local write "stop after"(w315) -> ()
          }
        }
        n233 = call <vilib>:"General Error Handler.vi"("error in (no error)"=w278) -> ()  [unwired: 10 in, 5 out]
      }
      frame "cont_scan" {
        n234 = Dequeue Element(queue=w418) -> ()  [unwired: 2 in, 4 out]
        n235 = Unbundle By Name(w403) -> ("DAC_cmd"=w402:refnum<queue>)
        n236 = Insert Into Array(array="delay_speedpoints", index (col)=1 ("disabled index (col)"), new element=string[] [] ("new element/subarray")) -> (w414:string[][])  [unwired: 1 in]
        n237 = Unbundle By Name(w403) -> ("ESP_cmd"=w388:refnum<queue>)
        n238 = Unbundle By Name(w413) -> ("ESP_data"=w412:refnum<queue>)
        n239 = call "create scan vectr2.1.vi"("Table Control"=w414) -> ("parameters"=w410:dbl[], "positions"=w411:dbl[])  [unwired: 3 in]
        n240 = Reverse 1D Array(array=w411) -> (reversed array=w405:dbl[])
        n241 = Reverse 1D Array(array=w410) -> (reversed array=w409:dbl[])
        n242 = local read "time_zero"() -> (w400:dbl)
        n243 = Index Array(array=w411) -> (element=w385:dbl)  [unwired: 1 in]
        n244 = Index Array(array=w405) -> (element=w399:dbl)  [unwired: 1 in]
        n245 = call "ESP_Q_abs.vi"("Position"=w385, "Axis"=w386, "queue"=w388) -> ("error out"=w389:errorcluster, "queue out"=w387:refnum<queue>)  [unwired: 7 in]
        n246 = call "time2mm001.vi"("Offset (mm)"=w400, "time"=w385) -> ("position (mm)"=w397:dbl)  [unwired: 1 in]
        n247 = call "time2mm001.vi"("Offset (mm)"=w400, "time"=w399) -> ("position (mm)"=w398:dbl)  [unwired: 1 in]
        n248 = call "wait4noti.vi"("error in (no error)"=w389, "notifier"=w392) -> ("error out"=w390:errorcluster, "notifier out"=w391:refnum<notifier>)  [unwired: 8 in]
        n249 = Format Into String(format string="cont:on:%6.6f:%6.6f", w397, w398) -> (resulting string=w401:string)  [unwired: 2 in, 1 out]
        n250 = call-poly <userlib>:"CaLabPut.vi"("Error in (no error)"=w390, "Values"=i32[] [0, 1, 1], "PV Names"=string[] ["SCDLD:cam1:Acquire", "SCDLD:cam1:ZeroCube", "SCDLD:cam1:RawEventDataStreamRestartFP"]) -> ("Error out"=w406:errorcluster)  [unwired: 5 in, 3 out]
        n251 = Enqueue Element(queue=w402, element=w401) -> (queue out=w396:refnum<queue>)  [unwired: 2 in, 2 out]
        n252 = while {
          tunnel: w412 -> [w445]
          tunnel: w400 -> [w444]
          tunnel: w391 -> [w443]
          tunnel: w386 -> [w428]
          shift-right: [w421] -> w394
          shift-left: w406 -> [w433]
          tunnel: w387 -> [w432]
          shift-right: [w437] -> _
          shift-left: w405 -> [w438]
          shift-right: [w436] -> _
          shift-left: w409 -> [w439]
          i -> [w442]
          stop <- w434 stop-if-true
          n253 = Reverse 1D Array(array=w439) -> (reversed array=w436:dbl[])
          n254 = Index Array(array=w436) -> (element=w431:dbl)  [unwired: 1 in]
          n255 = Index Array(array=w438) -> (element=w427:dbl)  [unwired: 1 in]
          n256 = Reverse 1D Array(array=w438) -> (reversed array=w437:dbl[])
          n257 = call "ESP_Q_vel.vi"("error in (no error)"=w433, "Position"=w431, "Axis"=w428, "queue"=w432) -> ("error out"=w429:errorcluster, "queue out"=w430:refnum<queue>)  [unwired: 6 in]
          n258 = call "ESP_Q_abs.vi"("error in (no error)"=w429, "Position"=w427, "Axis"=w428, "queue"=w430) -> ("error out"=w425:errorcluster, "queue out"=w426:refnum<queue>)  [unwired: 6 in]
          n259 = Quotient & Remainder(x=w442, y=2) -> (x-y*floor(x/y)=w441:i32)  [unwired: 1 out]
          n260 = Not Equal To 0?(x=w441) -> (x != 0?=w440:bool)
          n261 = for {
            tunnel: w436 -> [w451] mode=indexing
            tunnel: w426 -> [w453]
            tunnel: w437 -> [w460] mode=indexing
            tunnel: w445 -> [w461]
            tunnel: w444 -> [w459]
            tunnel: w443 -> [w457]
            tunnel: w428 -> [w452]
            tunnel: w440 -> [w456]
            shift-right: [w448] -> w423
            shift-left: w425 -> [w454]
            tunnel: [w449] -> w435
            stop <- w450 continue-if-true
            n262 = call "time2mm001.vi"("Offset (mm)"=w459, "time"=w460) -> ("position (mm)"=w458:dbl)  [unwired: 1 in]
            n263 = call "ESP_Q_vel.vi"("error in (no error)"=w454, "Position"=w451, "Axis"=w452, "queue"=w453) -> ("error out"=w455:errorcluster)  [unwired: 6 in, 1 out]
            n264 = while {
              tunnel: w461 -> [w480]
              tunnel: w458 -> [w474]
              tunnel: w457 -> [w476]
              tunnel: [w467] -> w450
              tunnel: w456 -> [w470]
              shift-right: [w466] -> w448
              shift-left: w455 -> [w478]
              tunnel: [w462] -> w449
              stop <- w475 continue-if-true
              n265 = local read "stop now"() -> (w462:bool)
              n266 = Preview Queue Element(queue=w480, timeout in ms (-1)=5000, error in (no error)=w478) -> (element=w479:T5, error out=w466:errorcluster)  [unwired: 2 out]
              n267 = Wait on Notification(notifier=w476, ignore previous (F)=TRUE) -> (notification=w468:bool)  [unwired: 2 in, 3 out]
              n268 = Unbundle(w479) -> ("Axis 1"=w473:dbl)  [unwired: 2 out]
              n269 = Less?(x=w474, y=w473) -> (x < y?=w472:bool)
              n270 = Greater?(x=w474, y=w473) -> (0:w471:bool)
              n271 = Select(t=w472, s=w470, f=w471) -> (s? t:f=w469:bool)
              n272 = Not(x=w466) -> (.not. x?=w464:bool)
              n273 = Not(x=w462) -> (.not. x?=w463:bool)
              n274 = Compound Arithmetic op=AND(w468, w464, w463) -> (w467:bool)
              n275 = Compound Arithmetic op=AND(w467, w469) -> (w475:bool)
            }
          }
          n276 = flat-sequence {
            tunnel: [w447] -> w422
            tunnel: w423 -> [w446]
            tunnel: [w446] -> w421
            frame #0 {
              n277 = local read "stop after"() -> (w447:bool)
            }
          }
          n278 = Compound Arithmetic op=OR(w435, w421, w422) -> (w434:bool)
        }
        n279 = flat-sequence {
          tunnel: w394 -> [w420]
          tunnel: [w420] -> w393
          frame #0 {
            w419 = FALSE
            n280 = local write "stop after"(w419) -> ()
            n281 = local write "stop now"(w419) -> ()
          }
        }
        n282 = Enqueue Element(queue=w396, element="cont:off" ("format string"), error in (no error)=w393) -> ()  [unwired: 1 in, 3 out]
      }
    }
  }
  n283 = while {
    tunnel: w42 -> [w500]
    tunnel: w35 -> [w493]
    shift-right: [w482] -> _
    shift-left: _ -> [w492]
    shift-right: [w491] -> _
    shift-left: _ -> [w489]
    shift-right: [w481] -> _
    shift-left: errorcluster {"status"=FALSE, "code"=0, "source"=""} ("error out") -> [w490]
    tunnel: w39 -> [w488]
    tunnel: w36 -> [w486]
    stop <- w494 stop-if-true
    # "ESP301"
    n284 = Preview Queue Element(queue=w500, timeout in ms (-1)=w492) -> (queue out=w495:refnum<queue>, element=w499:string)  [unwired: 1 in, 2 out]
    n285 = Match Pattern(string=w499, regular expression=":") -> (before substring=w497:string, after substring=w496:string)  [unwired: 1 in, 2 out]
    n286 = case shown="\"idle\", Default" w497 {
      tunnel: w496 -> [_ _ w564 w599 w631 w655 w685 _ _ _]
      tunnel: w495 -> [_ w542 w572 w606 w635 w666 w690 w721 w726 w738]
      tunnel: [_ _ _ _ _ _ _ TRUE _ _] -> w494
      tunnel: w493 -> [_ _ _ _ _ _ _ w714 _ _]
      tunnel: [0 0 0 0 0 0 0 0 -1 0] -> w483
      tunnel: [w518 w545 w558 w593 w624 w663 w695 w717 refnum<visa-resource-name> refnum ("VISA resource name out") w737] -> w491
      tunnel: [w516 w544 w567 w602 w623 w662 w694 w716 w725 w736] -> w481
      tunnel: w490 -> [w521 w546 w570 w604 w627 w664 w693 w716 w723 _]
      tunnel: w489 -> [w522 w547 w571 w605 w628 w665 w692 w717 w722 _]
      tunnel: w488 -> [w517 _ w566 w601 _ _ _ w711 _ _]
      tunnel: "ESP Patch" -> [w519 _ w561 w596 w630 w658 w688 _ _ _]
      tunnel: w486 -> [w520 _ _ _ _ _ _ _ _ _]
      tunnel: "time_zero" -> [w515 _ _ w589 _ _ _ _ _ _]
      frame "idle", Default {
        # "#ToDo combine to one command"
        n287 = Index Array(array=w519) -> (element #1=w513:i32, element #2=w512:i32, element #3=w511:i32)  [unwired: 3 in]
        n288 = disable-structure shown="Enabled" {
          disable-tunnel: w522 -> [w540 _]
          disable-tunnel: w521 -> [w539 _]
          disable-tunnel: [w538 _] -> w518
          disable-tunnel: w513 -> [w533 _]
          disable-tunnel: w512 -> [w532 _]
          disable-tunnel: w511 -> [w531 _]
          disable-tunnel: [w528 _] -> w510
          disable-tunnel: [w527 _] -> w505
          disable-tunnel: [w526 _] -> w504
          disable-tunnel: [w525 _] -> w502
          disable-tunnel: [w524 _] -> w501
          frame Enabled {
            n289 = call "Read Actual Position.vi"("error in (no error)"=w539, "Axis (1)"=w533, "VISA resource name"=w540) -> ("error out"=w536:errorcluster, "Position (units)"=w526:dbl, "VISA resource name out"=w537:refnum<visa-resource-name>)  [unwired: 2 in]
            n290 = call "Read Actual Position.vi"("error in (no error)"=w536, "Axis (1)"=w532, "VISA resource name"=w537) -> ("error out"=w534:errorcluster, "Position (units)"=w525:dbl, "VISA resource name out"=w535:refnum<visa-resource-name>)  [unwired: 2 in]
            n291 = call "Read Actual Position.vi"("error in (no error)"=w534, "Axis (1)"=w531, "VISA resource name"=w535) -> ("error out"=w529:errorcluster, "Position (units)"=w524:dbl, "VISA resource name out"=w530:refnum<visa-resource-name>)  [unwired: 2 in]
            n292 = call "Get Controller Status.vi"("error in (no error)"=w529, "VISA resource name"=w530) -> ("error out"=w527:errorcluster, "Controller Status"=w528:T9, "VISA resource name out"=w538:refnum<visa-resource-name>)  [unwired: 2 in, 1 out]
          }
          frame Disabled {
            n293 = Wait (ms)(milliseconds to wait=u32 100) -> ()  [unwired: 1 out]
          }
        }
        "delay_pos_mm" <- w504
        "pump_position" <- w502
        "probe_position" <- w501
        n294 = call "mm2time001.vi"("Offset (mm)"=w515, "distance (mm)"=w504) -> ("time in fs"=→"delay_pos_fs":dbl)  [unwired: 1 in]
        n295 = Bundle("Position (units)"=w504, "Position (units)"=w502, "Position (units)"=w501) -> (w514:T10)  [unwired: 1 in]
        n296 = Lossy Enqueue Element(queue=w520, element=w514) -> ()  [unwired: 1 in, 4 out]
        n297 = Unbundle(w510) -> ("Axis1 moving"=w507:bool, "Axis2 moving"=w508:bool, "Axis3 moving"=w509:bool)  [unwired: 13 out]
        n298 = Compound Arithmetic op=OR(w507, w508, w509) -> (w506:bool)
        n299 = Send Notification(notification=w506, notifier=w517, error in (no error)=w505) -> (error out=w516:errorcluster)  [unwired: 1 out]
      }
      frame "stop" {
        n300 = Dequeue Element(queue=w542) -> ()  [unwired: 2 in, 4 out]
        n301 = disable-structure shown="Enabled" {
          disable-tunnel: w547 -> [w552 _]
          disable-tunnel: w546 -> [w551 _]
          disable-tunnel: [w550 _] -> w545
          disable-tunnel: [w549 _] -> w544
          frame Enabled {
            n302 = call "Stop Motion.vi"("error in (no error)"=w551, "Stop all axes (F)"=TRUE, "VISA resource name"=w552) -> ("error out"=w549:errorcluster, "VISA resource name out"=w550:refnum<visa-resource-name>)  [unwired: 3 in]
          }
          frame Disabled {
            n303 = local read "String"() -> (w554:string)
            n304 = Concatenate Strings(w554, "ESP_stop_motion" ("string")) -> (w553:string)
            n305 = local write "String"(w553) -> ()
          }
        }
      }
      frame "abs" {
        n306 = Dequeue Element(queue=w572) -> ()  [unwired: 2 in, 4 out]
        n307 = Match Pattern(string=w564, regular expression=":") -> (before substring=w563:string, after substring=w562:string)  [unwired: 1 in, 2 out]
        n308 = Decimal String To Number(string=w563) -> (number=w559:i32)  [unwired: 2 in, 1 out]
        n309 = Fract/Exp String To Number(string=w562) -> (number=w569:dbl)  [unwired: 3 in, 1 out]
        n310 = Index Array(array=w561, index=w559) -> (element=w560:i32)
        n311 = disable-structure shown="Enabled" {
          disable-tunnel: w571 -> [w578 _]
          disable-tunnel: w570 -> [w577 _]
          disable-tunnel: w569 -> [w576 w581]
          disable-tunnel: w560 -> [w575 w584]
          disable-tunnel: [w574 _] -> w558
          disable-tunnel: [w573 _] -> w557
          frame Enabled {
            n312 = call "Move Absolute.vi"("error in (no error)"=w577, "Position (0 units)"=w576, "Axis (1)"=w575, "VISA resource name"=w578) -> ("error out"=w573:errorcluster, "VISA resource name out"=w574:refnum<visa-resource-name>)  [unwired: 2 in]
          }
          frame Disabled {
            n313 = Number To Fractional String(number=w581) -> (F-format string=w580:string)  [unwired: 3 in]
            n314 = Number To Decimal String(number=w584) -> (decimal integer string=w583:string)  [unwired: 1 in]
            n315 = local read "String"() -> (w586:string)
            n316 = Concatenate Strings(w586, "ESP_abs_axis:" ("string"), w583, "_value:" ("string"), w580, "\n" ("string")) -> (w585:string)
            n317 = local write "String"(w585) -> ()
          }
        }
        n318 = Send Notification(notification=TRUE, notifier=w566, error in (no error)=w557) -> (error out=w567:errorcluster)  [unwired: 1 out]
      }
      frame "absfs" {
        n319 = Dequeue Element(queue=w606) -> ()  [unwired: 2 in, 4 out]
        n320 = Match Pattern(string=w599, regular expression=":") -> (before substring=w598:string, after substring=w597:string)  [unwired: 1 in, 2 out]
        n321 = Decimal String To Number(string=w598) -> (number=w594:i32)  [unwired: 2 in, 1 out]
        n322 = Fract/Exp String To Number(string=w597) -> (number=w590:dbl)  [unwired: 3 in, 1 out]
        n323 = call "time2mm001.vi"("Offset (mm)"=w589, "time"=w590) -> ("position (mm)"=w588:dbl)  [unwired: 1 in]
        n324 = Index Array(array=w596, index=w594) -> (element=w595:i32)
        n325 = disable-structure shown="Enabled" {
          disable-tunnel: w605 -> [w612 _]
          disable-tunnel: w604 -> [w611 _]
          disable-tunnel: w595 -> [w610 w618]
          disable-tunnel: [w609 _] -> w593
          disable-tunnel: [w608 _] -> w592
          disable-tunnel: w588 -> [w607 w617]
          frame Enabled {
            n326 = call "Move Absolute.vi"("error in (no error)"=w611, "Position (0 units)"=w607, "Axis (1)"=w610, "VISA resource name"=w612) -> ("error out"=w608:errorcluster, "VISA resource name out"=w609:refnum<visa-resource-name>)  [unwired: 2 in]
          }
          frame Disabled {
            n327 = Number To Decimal String(number=w618) -> (decimal integer string=w616:string)  [unwired: 1 in]
            n328 = local read "String"() -> (w620:string)
            n329 = Number To Fractional String(number=w617) -> (F-format string=w614:string)  [unwired: 3 in]
            n330 = Concatenate Strings(w620, "ESP_absfs_axis:" ("string"), w616, "_value:" ("string"), w614, "\n" ("string")) -> (w619:string)
            n331 = local write "String"(w619) -> ()
          }
        }
        n332 = Send Notification(notification=TRUE, notifier=w601, error in (no error)=w592) -> (error out=w602:errorcluster)  [unwired: 1 out]
      }
      frame "rel" {
        n333 = Dequeue Element(queue=w635) -> ()  [unwired: 2 in, 4 out]
        n334 = Match Pattern(string=w631, regular expression=":") -> (before substring=w633:string, after substring=w634:string)  [unwired: 1 in, 2 out]
        n335 = Decimal String To Number(string=w633) -> (number=w629:i32)  [unwired: 2 in, 1 out]
        n336 = Fract/Exp String To Number(string=w634) -> (number=w625:dbl)  [unwired: 3 in, 1 out]
        n337 = Index Array(array=w630, index=w629) -> (element=w626:i32)
        n338 = disable-structure shown="Enabled" {
          disable-tunnel: w628 -> [w641 _]
          disable-tunnel: w627 -> [w640 _]
          disable-tunnel: w626 -> [w639 w647]
          disable-tunnel: w625 -> [w638 w646]
          disable-tunnel: [w637 _] -> w624
          disable-tunnel: [w636 _] -> w623
          frame Enabled {
            n339 = call "Move Relative.vi"("error in (no error)"=w640, "Position (0 units)"=w638, "Axis (1)"=w639, "VISA resource name"=w641) -> ("error out"=w636:errorcluster, "VISA resource name out"=w637:refnum<visa-resource-name>)  [unwired: 2 in]
          }
          frame Disabled {
            n340 = Number To Decimal String(number=w647) -> (decimal integer string=w645:string)  [unwired: 1 in]
            n341 = Number To Fractional String(number=w646) -> (F-format string=w643:string)  [unwired: 3 in]
            n342 = local read "String"() -> (w649:string)
            n343 = Concatenate Strings(w649, "ESP_rel_axis:" ("string"), w645, "_value:" ("string"), w643, "\n" ("string")) -> (w648:string)
            n344 = local write "String"(w648) -> ()
          }
        }
      }
      frame "relfs" {
        n345 = Dequeue Element(queue=w666) -> ()  [unwired: 2 in, 4 out]
        n346 = Match Pattern(string=w655, regular expression=":") -> (before substring=w653:string, after substring=w654:string)  [unwired: 1 in, 2 out]
        n347 = Decimal String To Number(string=w653) -> (number=w652:i32)  [unwired: 2 in, 1 out]
        n348 = Index Array(array=w658, index=w652) -> (element=w657:i32)
        n349 = Fract/Exp String To Number(string=w654) -> (number=w660:dbl)  [unwired: 3 in, 1 out]
        n350 = call "time2mm001.vi"("Offset (mm)"=0.0, "time"=w660) -> ("position (mm)"=w659:dbl)  [unwired: 1 in]
        n351 = disable-structure shown="Enabled" {
          disable-tunnel: w665 -> [w672 _]
          disable-tunnel: w664 -> [w671 _]
          disable-tunnel: [w670 _] -> w663
          disable-tunnel: [w669 _] -> w662
          disable-tunnel: w659 -> [w668 w677]
          disable-tunnel: w657 -> [w667 w678]
          frame Enabled {
            n352 = call "Move Relative.vi"("error in (no error)"=w671, "Position (0 units)"=w668, "Axis (1)"=w667, "VISA resource name"=w672) -> ("error out"=w669:errorcluster, "VISA resource name out"=w670:refnum<visa-resource-name>)  [unwired: 2 in]
          }
          frame Disabled {
            n353 = Number To Decimal String(number=w678) -> (decimal integer string=w676:string)  [unwired: 1 in]
            n354 = Number To Fractional String(number=w677) -> (F-format string=w675:string)  [unwired: 3 in]
            n355 = local read "String"() -> (w680:string)
            n356 = Concatenate Strings(w680, "ESP_relfs_axis:" ("string"), w676, "_value:" ("string"), w675, "\n" ("string")) -> (w679:string)
            n357 = local write "String"(w679) -> ()
          }
        }
      }
      frame "vel" {
        n358 = Dequeue Element(queue=w690) -> ()  [unwired: 2 in, 4 out]
        n359 = Match Pattern(string=w685, regular expression=":") -> (before substring=w683:string, after substring=w684:string)  [unwired: 1 in, 2 out]
        n360 = Decimal String To Number(string=w683) -> (number=w682:i32)  [unwired: 2 in, 1 out]
        n361 = Fract/Exp String To Number(string=w684) -> (number=w691:dbl)  [unwired: 3 in, 1 out]
        n362 = Index Array(array=w688, index=w682) -> (element=w687:i32)
        n363 = disable-structure shown="Enabled" {
          disable-tunnel: [w701 _] -> w695
          disable-tunnel: [w700 _] -> w694
          disable-tunnel: w693 -> [w699 _]
          disable-tunnel: w692 -> [w698 _]
          disable-tunnel: w691 -> [w697 w706]
          disable-tunnel: w687 -> [w696 w707]
          frame Enabled {
            n364 = call "Set Velocity.vi"("error in (no error)"=w699, "Velocity (units/s)"=w697, "Axis (1)"=w696, "VISA resource name"=w698) -> ("error out"=w700:errorcluster, "VISA resource name out"=w701:refnum<visa-resource-name>)  [unwired: 2 in]
          }
          frame Disabled {
            n365 = Number To Fractional String(number=w706) -> (F-format string=w704:string)  [unwired: 3 in]
            n366 = Number To Decimal String(number=w707) -> (decimal integer string=w705:string)  [unwired: 1 in]
            n367 = local read "String"() -> (w710:string)
            n368 = Concatenate Strings(w710, "ESP_vel_axis:" ("string"), w705, "_value:" ("string"), w704, "\n" ("string")) -> (w709:string)
            n369 = local write "String"(w709) -> ()
          }
        }
      }
      frame "close" {
        n370 = Dequeue Element(queue=w721) -> (queue out=w720:refnum<queue>, error out=w719:errorcluster)  [unwired: 2 in, 2 out]
        n371 = Release Notifier(notifier=w711) -> ()  [unwired: 2 in, 3 out]
        n372 = Unbundle By Name(w714) -> ("ESP_data"=w712:refnum<queue>)
        n373 = Release Queue(queue=w720, error in (no error)=w719) -> ()  [unwired: 1 in, 3 out]
        n374 = Flush Queue(queue=w712) -> (queue out=w713:refnum<queue>)  [unwired: 1 in, 2 out]
        n375 = Release Queue(queue=w713) -> ()  [unwired: 2 in, 3 out]
      }
      frame "release" {
        n376 = Dequeue Element(queue=w726) -> ()  [unwired: 2 in, 4 out]
        n377 = disable-structure shown="Enabled" {
          disable-tunnel: [w732 _] -> w725
          disable-tunnel: w723 -> [w731 _]
          disable-tunnel: w722 -> [w728 _]
          frame Enabled {
            n378 = call "Stop Motion.vi"("error in (no error)"=w731, "VISA resource name"=w728) -> ("error out"=w730:errorcluster, "VISA resource name out"=w729:refnum<visa-resource-name>)  [unwired: 4 in]
            n379 = call "Close.vi"("error in (no error)"=w730, "VISA resource name"=w729) -> ("error out"=w732:errorcluster)  [unwired: 9 in]
          }
          frame Disabled {
            n380 = local read "String"() -> (w735:string)
            n381 = Concatenate Strings(w735, "ESP_release\n" ("string")) -> (w734:string)
            n382 = local write "String"(w734) -> ()
          }
        }
      }
      frame "initialize" {
        n383 = Dequeue Element(queue=w738) -> ()  [unwired: 2 in, 4 out]
        n384 = disable-structure shown="Enabled" {
          disable-tunnel: [w743 _] -> w737
          disable-tunnel: [w742 _] -> w736
          frame Enabled {
            n385 = call "Initialize.vi"("VISA resource name"="ESP301 COM PORT", "error in (no error)"=errorcluster {"status"=FALSE, "code"=0, "source"=""}, "Serial Link (RS232)"="Serial Link (RS232)") -> ("VISA resource name out"=w745:refnum<visa-resource-name>, "error out"=w744:errorcluster)  [unwired: 6 in]
            n386 = call "Get Velocity.vi"("error in (no error)"=w744, "VISA resource name"=w745) -> ("error out"=w742:errorcluster, "Velocity (units/s)"=w741:dbl, "VISA resource name out"=w743:refnum<visa-resource-name>)  [unwired: 3 in]
            n387 = local write "delay_velocity"(w741) -> ()
          }
          frame Disabled {
            n388 = local read "String"() -> (w750:string)
            n389 = Concatenate Strings(w750, "ESP_init\n" ("string")) -> (w749:string)
            n390 = local write "String"(w749) -> ()
          }
        }
      }
    }
    "ESP error" <- w481
    n391 = Select(t=-1, s=w481, f=w483) -> (s? t:f=w482:i32)
  }
  n392 = while {
    shift-right: [w751] -> _
    shift-left: _ -> [w771]
    shift-right: [w753] -> _
    shift-left: _ -> [w770]
    tunnel: w38 -> [w769]
    shift-right: [w768] -> _
    shift-left: _ -> [w767]
    tunnel: w37 -> [w766]
    tunnel: w35 -> [w765]
    shift-right: [w764] -> _
    shift-left: _ -> [w763]
    shift-right: [w760] -> _
    shift-left: w34 -> [w762]
    shift-right: [w759] -> _
    shift-left: w33 -> [w761]
    shift-right: [w757] -> _
    shift-left: w32 -> [w758]
    shift-right: [w756] -> _
    shift-left: _ -> [w755]
    stop <- w772 stop-if-true
    n393 = Preview Queue Element(queue=w769, timeout in ms (-1)=w771) -> (queue out=w773:refnum<queue>, element=w777:string)  [unwired: 1 in, 2 out]
    n394 = Match Pattern(string=w777, regular expression=":") -> (before substring=w775:string, after substring=w774:string)  [unwired: 1 in, 2 out]
    n395 = case shown="\"idle\", Default" w775 {
      tunnel: w774 -> [_ w841 _ _ _ _]
      tunnel: w773 -> [_ w829 w862 w889 w899 w922]
      tunnel: [_ _ _ TRUE _ _] -> w772
      tunnel: [0 _ _ _ -1 0] -> w752
      tunnel: [w786 w835 w861 w885 w890 w921] -> w753
      tunnel: w770 -> [w784 w835 w858 w885 w897 w920]
      tunnel: [w787 w836 w857 w884 w895 w923] -> w768
      tunnel: w767 -> [w785 w836 w857 w884 w898 _]
      tunnel: w766 -> [w788 _ _ _ _ _]
      tunnel: w765 -> [_ _ _ w881 _ _]
      tunnel: [w783 w834 w859 w880 w895 w915] -> w764
      tunnel: w763 -> [w783 w834 w860 w880 w896 _]
      tunnel: w762 -> [w782 w833 w856 w879 w894 w919]
      tunnel: w761 -> [w781 w832 w855 w878 w893 w918]
      tunnel: [w782 w827 w856 w879 w894 w919] -> w760
      tunnel: [w781 w826 w855 w878 w893 w918] -> w759
      tunnel: w758 -> [w780 w831 w854 w877 w892 w917]
      tunnel: [w780 w830 w854 w877 w892 w917] -> w757
      tunnel: [w778 w828 w853 w876 w891 w916] -> w756
      tunnel: w755 -> [w779 w828 w853 w876 w891 w916]
      frame "idle", Default {
        n396 = disable-structure shown="Enabled" {
          disable-tunnel: w788 -> [w806 _]
          disable-tunnel: [w805 _] -> w787
          disable-tunnel: [w804 _] -> w786
          disable-tunnel: w785 -> [w803 _]
          disable-tunnel: w784 -> [w802 _]
          disable-tunnel: w782 -> [w800 _]
          disable-tunnel: w781 -> [w799 _]
          disable-tunnel: w780 -> [w796 _]
          disable-tunnel: w779 -> [w793 _]
          disable-tunnel: [w792 _] -> w778
          frame Enabled {
            n397 = call <vilib>:"High Resolution Relative Seconds.vi"() -> ("relative seconds"=w790:dbl)
            n398 = Preview Queue Element(queue=w806, timeout in ms (-1)=0) -> (element=w801:T5, timed out?=w794:bool)  [unwired: 1 in, 2 out]
            n399 = case shown="False" w794 {
              tunnel: w801 -> [w813 _]
              tunnel: [w809 w814] -> w792
              tunnel: w793 -> [_ w814]
              tunnel: w790 -> [w808 _]
              frame False {
                n400 = Unbundle(w813) -> ("Axis 1"=w811:dbl)  [unwired: 2 out]
                n401 = call <vilib>:"General Polynomial Fit PtByPt.vi"("sample length"=10, "polynomial order"=3, "x"=w808, "y"=w811) -> ("Polynomial Fit Coefficients"=w809:dbl[])  [unwired: 2 in, 3 out]
              }
              frame True {
              }
            }
            n402 = call <vilib>:"1D Polynomial Evaluation PtByPt.vi"("Coefficients: a"=w792, "x"=w790) -> ("y"=w791:dbl)
            n403 = In Range and Coerce(upper limit=w800, x=w791, lower limit=w799) -> (In Range?=w797:bool)  [unwired: 1 out]
            n404 = And(x=w797, y=w796) -> (x .and. y?=w795:bool)
            n405 = case shown="False" w795 {
              tunnel: w791 -> [_ w819]
              tunnel: w800 -> [_ w818]
              tunnel: w799 -> [_ w817]
              tunnel: [3.0 ("DAC_Voutput") w816] -> w798
              frame False {
              }
              frame True {
                n406 = Subtract(x=w819, y=w818) -> (x-y=w824:dbl)
                n407 = Subtract(x=w818, y=w817) -> (x-y=w823:dbl)
                n408 = Divide(x=w824, y=w823) -> (x/y=w822:dbl)
                n409 = Increment(x=w822) -> (x+1=w821:dbl)
                n410 = Multiply(x=w821, y=8.0) -> (x*y=w816:dbl)
              }
            }
            "DAC_Voutput" <- w798
            n411 = call-poly <vilib>:"DAQmx Write.vi"("task/channels in"=w803, "data"=w798, "error in"=w802) -> ("task out"=w805:refnum<k21>, "error out"=w804:errorcluster)  [unwired: 10 in, 1 out]
          }
          frame Disabled {
            n412 = Wait (ms)(milliseconds to wait=u32 100) -> ()  [unwired: 1 out]
          }
        }
      }
      frame "cont" {
        n413 = Dequeue Element(queue=w829) -> ()  [unwired: 2 in, 4 out]
        n414 = Match Pattern(string=w841, regular expression=":") -> (before substring=w840:string, after substring=w837:string)  [unwired: 1 in, 2 out]
        n415 = Equal?(x="on", y=w840) -> (x = y?=w838:bool)
        n416 = case shown="True" w838 {
          tunnel: w837 -> [_ w851]
          tunnel: w833 -> [w844 _]
          tunnel: w832 -> [w843 _]
          tunnel: w831 -> [_ _]
          tunnel: [w844 w848] -> w827
          tunnel: [w843 w847] -> w826
          tunnel: [FALSE TRUE] -> w830
          frame False {
          }
          frame True {
            n417 = Match Pattern(string=w851, regular expression=":") -> (before substring=w850:string, after substring=w849:string)  [unwired: 1 in, 2 out]
            n418 = Fract/Exp String To Number(string=w849) -> (number=w847:dbl)  [unwired: 3 in, 1 out]
            n419 = Fract/Exp String To Number(string=w850) -> (number=w848:dbl)  [unwired: 3 in, 1 out]
          }
        }
      }
      frame "pulse" {
        n420 = Dequeue Element(queue=w862) -> ()  [unwired: 2 in, 4 out]
        n421 = disable-structure shown="Enabled" {
          disable-tunnel: [w866 _] -> w861
          disable-tunnel: w860 -> [w865 _]
          disable-tunnel: [w864 _] -> w859
          disable-tunnel: w858 -> [w863 _]
          frame Enabled {
            n422 = call-poly <vilib>:"DAQmx Write.vi"("task/channels in"=w865, "data"=6.0, "error in"=w863) -> ("task out"=w869:refnum<k21>, "error out"=w872:errorcluster)  [unwired: 10 in, 1 out]
            n423 = call "700a36db-ce49-4288-8972-970908bb0277.vi"("value in"=w872, "milliseconds to wait"=u32 3) -> ("value out"=w870:errorcluster)  [unwired: 1 out]
            n424 = call-poly <vilib>:"DAQmx Write.vi"("task/channels in"=w869, "data"=0.0, "error in"=w870) -> ("task out"=w864:refnum<k21>, "error out"=w866:errorcluster)  [unwired: 10 in, 1 out]
          }
          frame Disabled {
            n425 = local read "String"() -> (w874:string)
            n426 = Concatenate Strings(w874, "DAC_pulse\n" ("string")) -> (w873:string)
            n427 = local write "String"(w873) -> ()
          }
        }
      }
      frame "close" {
        n428 = Unbundle By Name(w881) -> ("dev2_data"=w882:refnum<queue>)
        n429 = Flush Queue(queue=w882) -> (queue out=w883:refnum<queue>)  [unwired: 1 in, 2 out]
        n430 = Dequeue Element(queue=w889) -> (queue out=w888:refnum<queue>, error out=w887:errorcluster)  [unwired: 2 in, 2 out]
        n431 = Release Queue(queue=w883) -> ()  [unwired: 2 in, 3 out]
        n432 = Release Queue(queue=w888, error in (no error)=w887) -> ()  [unwired: 1 in, 3 out]
      }
      frame "release" {
        w895 = refnum<k21> refnum ("task out")
        n433 = Dequeue Element(queue=w899) -> ()  [unwired: 2 in, 4 out]
        n434 = disable-structure shown="Enabled" {
          disable-tunnel: w898 -> [w910 _]
          disable-tunnel: w897 -> [w905 _]
          disable-tunnel: w896 -> [w904 _]
          disable-tunnel: [w901 _] -> w890
          frame Enabled {
            n435 = call <vilib>:"DAQmx Stop Task.vi"("task/channels in"=w910, "error in"=w905) -> ("task out"=w909:refnum<k21>, "error out"=w908:errorcluster)  [unwired: 12 in]
            n436 = call <vilib>:"DAQmx Stop Task.vi"("task/channels in"=w904, "error in"=w905) -> ("task out"=w906:refnum<k21>, "error out"=w907:errorcluster)  [unwired: 12 in]
            n437 = call <vilib>:"DAQmx Clear Task.vi"("task in"=w909, "error in"=w908) -> ("error out"=w903:errorcluster)  [unwired: 13 in]
            n438 = call <vilib>:"DAQmx Clear Task.vi"("task in"=w906, "error in"=w907) -> ("error out"=w902:errorcluster)  [unwired: 13 in]
            n439 = Merge Errors(w903, w902) -> (w901:errorcluster)
          }
          frame Disabled {
            n440 = local read "String"() -> (w912:string)
            n441 = Concatenate Strings(w912, "DAC_release\n" ("string")) -> (w911:string)
            n442 = local write "String"(w911) -> ()
          }
        }
      }
      frame "initialize" {
        n443 = Dequeue Element(queue=w922) -> ()  [unwired: 2 in, 4 out]
        n444 = disable-structure shown="Enabled" {
          disable-tunnel: [w937 _] -> w923
          disable-tunnel: [w929 _] -> w921
          disable-tunnel: w920 -> [w925 _]
          disable-tunnel: [w924 _] -> w915
          frame Enabled {
            w926 = -1 items=["Default"=-1, "RSE"=10083, "Differential"=10106, "Pseudodifferential"=12529] ("output terminal configuration")
            w939 = -1 items=["Default"=-1, "RSE"=10083, "Differential"=10106, "Pseudodifferential"=12529] ("output terminal configuration")
            n445 = call-poly <vilib>:"DAQmx Create Virtual Channel.vi"("maximum value"=10.0, "minimum value"=0.0, "output terminal configuration"=w939, "physical channels"="toADC", "error in"=w925) -> ("task out"=w935:refnum<k21>, "error out"=w938:errorcluster)  [unwired: 9 in]
            n446 = call-poly <vilib>:"DAQmx Create Virtual Channel.vi"("maximum value"=10.0, "minimum value"=0.0, "output terminal configuration"=w926, "physical channels"="toMRC", "error in"=w925) -> ("task out"=w934:refnum<k21>, "error out"=w933:errorcluster)  [unwired: 9 in]
            n447 = call <vilib>:"DAQmx Start Task.vi"("task/channels in"=w934, "error in"=w933) -> ("task out"=w924:refnum<k21>, "error out"=w928:errorcluster)  [unwired: 12 in]
            n448 = call <vilib>:"DAQmx Start Task.vi"("task/channels in"=w935, "error in"=w938) -> ("task out"=w937:refnum<k21>, "error out"=w930:errorcluster)  [unwired: 12 in]
            n449 = Merge Errors(w930, w928) -> (w929:errorcluster)
          }
          frame Disabled {
            n450 = local read "String"() -> (w943:string)
            n451 = Concatenate Strings(w943, "DAC_init\n" ("string")) -> (w942:string)
            n452 = local write "String"(w942) -> ()
          }
        }
      }
    }
    "DAC error" <- w753
    n453 = Select(t=-1, s=w753, f=w752) -> (s? t:f=w751:i32)
  }
  n454 = while {
    tunnel: w30 -> [w956]
    shift-right: [w948] -> _
    shift-left: _ -> [w954]
    tunnel: w29 -> [w953]
    shift-right: [w952] -> _
    shift-left: _ -> [w951]
    shift-right: [w946] -> _
    shift-left: _ -> [w950]
    stop <- w955 stop-if-true
    # "mirr"
    n455 = Preview Queue Element(queue=w956, timeout in ms (-1)=w954) -> (queue out=w959:refnum<queue>, element=w960:string)  [unwired: 1 in, 2 out]
    n456 = Match Pattern(string=w960, regular expression=":") -> (before substring=w958:string, after substring=w957:string)  [unwired: 1 in, 2 out]
    n457 = case shown="\"idle\", Default" w958 {
      tunnel: w959 -> [w977 w1009 w1040 w1050 w1053 w1057 _]
      tunnel: w957 -> [w969 w1010 _ _ _ _ _]
      tunnel: [_ _ _ TRUE _ _ _] -> w955
      tunnel: [_ _ _ _ -1 _ _] -> w947
      tunnel: w953 -> [w966 _ _ w1046 _ _ _]
      tunnel: [w971 w1006 refnum<visa-resource-name> refnum ("VISA resource name out") w1048 w1052 w1056 w1066] -> w952
      tunnel: w951 -> [w976 w1008 w1039 w1048 w1052 _ w1068]
      tunnel: [w965 w1005 w1038 w1047 w1051 w1055 w1065] -> w946
      tunnel: w950 -> [w975 w1007 _ w1047 w1051 _ w1067]
      tunnel: "zaber_patch" -> [w964 w1004 _ _ _ _ w1064]
      frame "abs" {
        n458 = Dequeue Element(queue=w977) -> ()  [unwired: 2 in, 4 out]
        n459 = Scan From String(format string="%d:%f:%s", input string=w969) -> (output 1=w963:i32, output 2=w972:dbl, output 3=w970:string)  [unwired: 5 in, 3 out]
        n460 = Index Array(array=w964, index=w963) -> (element=w962:u8)
        n461 = disable-structure shown="Enabled" {
          disable-tunnel: w976 -> [w993 _]
          disable-tunnel: w975 -> [w992 _]
          disable-tunnel: w964 -> [_ _]
          disable-tunnel: w962 -> [w983 w999]
          disable-tunnel: w972 -> [w988 w998]
          disable-tunnel: [w985 _] -> w971
          disable-tunnel: [w984 _] -> w967
          frame Enabled {
            w991 = u8 20 items=["Echo"=55, "Home"=1, "Move Absolute"=20, "Move Relative"=21, "Move at Constant Speed"=22, "Renumber"=2, "Restore Settings"=36, "Stop"=23] ("Command")
            # "#ToDo does read pos wait for completion of movement?"
            n462 = Bundle("mirr_X# 4"=w983, "Command"=w991, w988, "Response Count"=1) -> (w989:T11)  [unwired: 1 in]
            n463 = call "Request Command.vi"("error in (no error)"=w992, "Request"=w989, "VISA resource name"=w993) -> ("error out"=w986:errorcluster, "VISA resource name out"=w987:refnum<visa-resource-name>)  [unwired: 5 in, 2 out]
            n464 = call "zaber_readpos.vi"("error in (no error)"=w986, "axis"=w983, "VISA in"=w987) -> ("error out"=w984:errorcluster, "VISA out"=w985:refnum<visa-resource-name>)  [unwired: 6 in, 1 out]
          }
          frame Disabled {
            n465 = local read "String"() -> (w1002:string)
            n466 = Number To Decimal String(number=w999) -> (decimal integer string=w997:string)  [unwired: 1 in]
            n467 = Number To Fractional String(number=w998) -> (F-format string=w996:string)  [unwired: 3 in]
            n468 = Concatenate Strings(w1002, "ZABER_abs_axis:" ("string"), w997, "_value:" ("string"), w996, "\n" ("string")) -> (w1001:string)
            n469 = local write "String"(w1001) -> ()
          }
        }
        n470 = Equal?(x=w970, y="wait") -> (x = y?=w968:bool)
        n471 = case shown="True" w968 {
          tunnel: w967 -> [w978 w982]
          tunnel: [w978 w981] -> w965
          tunnel: w966 -> [_ w980]
          frame False {
          }
          frame True {
            n472 = Send Notification(notification=TRUE, notifier=w980, error in (no error)=w982) -> (error out=w981:errorcluster)  [unwired: 1 out]
          }
        }
      }
      frame "rel" {
        n473 = Dequeue Element(queue=w1009) -> ()  [unwired: 2 in, 4 out]
        n474 = Match Pattern(string=w1010, regular expression=":") -> (before substring=w1012:string, after substring=w1011:string)  [unwired: 1 in, 2 out]
        n475 = Decimal String To Number(string=w1012) -> (number=w1003:i32)  [unwired: 2 in, 1 out]
        n476 = Decimal String To Number(string=w1011) -> (number=w1014:i32)  [unwired: 2 in, 1 out]
        n477 = disable-structure shown="Enabled" {
          disable-tunnel: w1014 -> [w1025 w1030]
          disable-tunnel: w1008 -> [w1021 _]
          disable-tunnel: w1007 -> [w1020 _]
          disable-tunnel: [w1019 _] -> w1006
          disable-tunnel: [w1018 _] -> w1005
          disable-tunnel: w1004 -> [w1017 _]
          disable-tunnel: w1003 -> [w1016 w1031]
          frame Enabled {
            w1024 = u8 21 items=["Echo"=55, "Home"=1, "Move Absolute"=20, "Move Relative"=21, "Move at Constant Speed"=22, "Renumber"=2, "Restore Settings"=36, "Stop"=23] ("Command")
            n478 = Index Array(array=w1017, index=w1016) -> (element=w1015:u8)
            n479 = Bundle("mirr_X# 4"=w1015, "Command"=w1024, w1025, "Response Count"=1) -> (w1022:T12)  [unwired: 1 in]
            n480 = call "Request Command.vi"("error in (no error)"=w1020, "Request"=w1022, "VISA resource name"=w1021) -> ("error out"=w1018:errorcluster, "VISA resource name out"=w1019:refnum<visa-resource-name>)  [unwired: 5 in, 2 out]
          }
          frame Disabled {
            n481 = Number To Decimal String(number=w1031) -> (decimal integer string=w1029:string)  [unwired: 1 in]
            n482 = Number To Decimal String(number=w1030) -> (decimal integer string=w1027:string)  [unwired: 1 in]
            n483 = local read "String"() -> (w1034:string)
            n484 = Concatenate Strings(w1034, "ZABER_rel_axis:" ("string"), w1029, "_value:" ("string"), w1027, "\n" ("string")) -> (w1033:string)
            n485 = local write "String"(w1033) -> ()
          }
        }
      }
      frame "release" {
        n486 = Dequeue Element(queue=w1040) -> (queue out=w1036:refnum<queue>)  [unwired: 2 in, 3 out]
        n487 = Enqueue Element(queue=w1036, element="suspend") -> ()  [unwired: 2 in, 3 out]
        n488 = disable-structure shown="Enabled" {
          disable-tunnel: w1039 -> [w1042 _]
          disable-tunnel: [w1041 _] -> w1038
          frame Enabled {
            n489 = call "Close.vi"("VISA resource name"=w1042) -> ("error out"=w1041:errorcluster)  [unwired: 9 in, 1 out]
          }
          frame Disabled {
            n490 = local read "String"() -> (w1044:string)
            n491 = Concatenate Strings(w1044, "ZABER_release\n" ("string")) -> (w1043:string)
            n492 = local write "String"(w1043) -> ()
          }
        }
      }
      frame "close" {
        n493 = Release Queue(queue=w1050) -> ()  [unwired: 2 in, 3 out]
        n494 = Release Notifier(notifier=w1046) -> ()  [unwired: 2 in, 3 out]
      }
      frame "suspend" {
        n495 = Dequeue Element(queue=w1053) -> ()  [unwired: 2 in, 4 out]
      }
      frame "initialize" {
        n496 = Dequeue Element(queue=w1057) -> ()  [unwired: 2 in, 4 out]
        n497 = disable-structure shown="Enabled" {
          disable-tunnel: [w1060 _] -> w1056
          disable-tunnel: [w1059 _] -> w1055
          frame Enabled {
            n498 = call "Initialize.vi"("VISA resource name"="zaber_VISA") -> ("error out"=w1059:errorcluster, "VISA resource name out"=w1060:refnum<visa-resource-name>)  [unwired: 8 in, 1 out]
          }
          frame Disabled {
            n499 = local read "String"() -> (w1063:string)
            n500 = Concatenate Strings(w1063, "ZABER_init\n" ("string")) -> (w1062:string)
            n501 = local write "String"(w1062) -> ()
          }
        }
      }
      frame "idle", Default {
        n502 = disable-structure shown="Enabled" {
          disable-tunnel: w1068 -> [w1079 _]
          disable-tunnel: w1067 -> [w1078 _]
          disable-tunnel: [w1075 _] -> w1066
          disable-tunnel: [w1074 _] -> w1065
          disable-tunnel: w1064 -> [w1071 _]
          frame Enabled {
            n503 = Index Array(array=w1071) -> (element #1=w1070:u8, element #2=w1069:u8)  [unwired: 2 in]
            n504 = call "zaber_readpos.vi"("error in (no error)"=w1078, "axis"=w1070, "VISA in"=w1079) -> ("error out"=w1076:errorcluster, "position"=→"zaber_Xpos":i32, "VISA out"=w1077:refnum<visa-resource-name>)  [unwired: 6 in]
            n505 = call "zaber_readpos.vi"("error in (no error)"=w1076, "axis"=w1069, "VISA in"=w1077) -> ("error out"=w1074:errorcluster, "position"=→"zaber_Ypos":i32, "VISA out"=w1075:refnum<visa-resource-name>)  [unwired: 6 in]
          }
          frame Disabled {
            n506 = Wait (ms)(milliseconds to wait=u32 100) -> ()  [unwired: 1 out]
          }
        }
      }
    }
    "zaber_error" <- w946
    n507 = Select(t=-1, s=w946, f=w947) -> (s? t:f=w948:i32)
  }
  n508 = disable-structure shown="Disabled" {
    frame Disabled {
      n509 = property on="Intensity Graph" class="IntGraph (strict)"("ActXScl"=0 ("Active X Scale")) -> ("XScale.Minimum"=w1084:dbl, "XScale.Maximum"=w1081:dbl)  [unwired: 2 in, 2 out]
      n510 = Multiply() -> (x*y=w1086:dbl)  [unwired: 2 in]
      n511 = Multiply(y=w1084) -> (x*y=w1083:dbl)  [unwired: 1 in]
      n512 = Multiply(y=w1081) -> (x*y=w1082:dbl)  [unwired: 1 in]
      n513 = property on="Intensity Graph" class="IntGraph (strict)" props=["ActXScl", "XScale", "Multiplier", "XScale", "Offset", "XScale", "Minimum", "XScale", "Maximum"]("ActXScl"=1 ("Active X Scale"), "XScale.Offset"=w1086, "XScale.Minimum"=w1083, "XScale.Maximum"=w1082) -> ()  [unwired: 3 in, 2 out]
    }
    frame Enabled {
    }
  }
